vi "Mixed Mode Widget.vi"() -> ()   [LabVIEW 2009]
uses:
  lib/MixedMode/Mixed Mode Command Action.ctl
  lib/MixedMode/Target Data.ctl
  lib/MixedMode/Ramp Time Tuple.ctl
  lib/MixedMode/Messages/Mixed Mode Command.ctl
  lib/MixedMode/Mixed Mode Cartesian Data.ctl
  lib/MixedMode/Mixed Mode Convergence Status.ctl
  lib/MixedMode/Mixed Mode States.ctl
  lib/MixedMode/Messages/Mixed Mode Status.ctl
  lib/MixedMode Widget/Mixed Mode Widget Button States.ctl
  lib/MixedMode/Step DAO Actions.ctl
  lib/MixedMode Widget/NTCP MM Requests.ctl
  lib/MixedMode/Messages/Mixed Mode Button Events.ctl
  lib/Data Access Objects/Metadata/LBCB Number.ctl
  lib/MixedMode/Messages/Target.ctl
  lib/MixedMode/Messages/Mixed Mode Button Events Message.ctl
  lib/MixedMode/Messages/MM Widget Parameter Changes.ctl
  lib/Apps/GUI Control.ctl
  lib/MixedMode/Messages/Mixed Mode GUI Update Type.ctl
  lib/MixedMode/Messages/Mixed Mode Gui Update Msg.ctl
  lib/Global Data/Names/Name Actions.ctl
  lib/MixedMode/MCL States.ctl
  lib/MixedMode Widget/Manual States.ctl
  lib/MixedMode Widget/Input File Step Actions.ctl
  lib/MixedMode Widget/Input File States.ctl
  lib/Apps/Yes No Button.ctl
  NTCP library/NTCP Commands.ctl
  lib/NTCP Client/MM 2 NTCP Message.ctl
  lib/NTCP Client/NTCP 2 MM Message.ctl
  lib/Data Access Objects/Metadata/Persistant DAO Actions.ctl
  lib/MixedMode Widget/NTCP Mixed Mode States.ctl
  lib/Launcher/Launcher Actions.ctl
  lib/Launcher/NoPanelAppTypes.ctl
  lib/MixedMode Widget/Skip NTCP Close Monitor.ctl
  lib/MixedMode Widget/Run Or Stop Result.ctl
  lib/Apps/On Off Button.ctl
  lib/MixedMode Widget/Blinkies.ctl
  lib/Data Access Objects/Metadata/DAO Actions.ctl
  lib/MixedMode/Mixed Mode Archived State.ctl
  lib/IPC Messages/Offset Message Type.ctl
  lib/MixedMode Widget/Mixed Mode State Display.ctl
  lib/MixedMode Widget/Target Pattern.ctl
  lib/Data Display/External Sensor Name & Value.ctl
panel:
  out "Force Tag":string
  in  "Force Tags":string[](array[string])
  out "Typo Problem":bool
  out "Increment Limit":bool caption="Increment"
  out "From Queue":string
  out "To Queue":string
  out "NTCP":T1
  out "MCL States":T5
  out "NTCP MM Requests":T6
  out "Force Limit":bool caption="Force"
  out "Displacement Limit":bool caption="Displacement"
  out "Messages":string
  out "Mixed Mode Status":T7={"LBCB Target"=[], "MixedModeStates"=enum."Idle", "LBCB Convergence"=[], "LBCB Measurements"=[]}
  in  "App Running":bool
  out "Button States":T12
  in  "App Stop":bool
  out "Mixed Mode Command":T13
  in  "Cartesian Type":bool caption="CartesianType"
  in  "Channel Data Tables":T16(tab)
  in  "LBCB 2 Label":string="LBCB 2"
  out "Cartesian Labels L1":string[](array[string])=["X", "Y", "Z", "Rx", "Ry", "Rz"]
  out "LBCB 1 Cartesian Space":dbl[][](array[numeric]) caption="LBCB 1"
  out "LBCB 2 Cartesian Space":dbl[][](array[numeric]) caption="LBCB 2"
  out "Cartesian Labels L2":string[](array[string])=["X", "Y", "Z", "Rx", "Ry", "Rz"]
  out "Cartesian Space Labels":string[](array[string])=["Commands (in/rad)", "Displacements (in/rad)", "Forces (lbs/lb*in)"]
  in  "LBCB 1 Label":string="LBCB 1"
  out "Actuator Labels L2":string[](array[string])=["X1", "X2", "Y1", "Z1", "Z2", "Z3"]
  out "LBCB 2 Actuator Space":dbl[][](array[numeric]) caption="LBCB 2"
  out "LBCB 1 Actuator Space":dbl[][](array[numeric]) caption="LBCB 1"
  out "Actuator Labels L1":string[](array[string])=["X1", "X2", "Y1", "Z1", "Z2", "Z3"]
  out "Actuator Space Labels":string[](array[string])=["Commands (in)", "Displacements (in)", "Forces (lbs)", "Integral"]
  out "External Sensors":T17[](array[typedef])
  out "Test Statistics":cluster{"Steps":string, "Elapsed \nTime":dbl} {"Elapsed \nTime" format="%<%H:%M:%S>t"}
  in  "Mixed Mode Control Tabs":enum32{"Manual", "Input File", "NTCP"}(tab)
  in  "Set Target":bool
  in  "Target Pattern":T18
  in  "Apply Pattern":bool
  out "Manual States":T19
  in  "Run Infile":bool
  out "Running":bool
  in  "Reset":bool
  in  "Load File":bool
  out "Input File States":T20
  in  "Connect Server":bool
  in  "Control Point":string="MDL-00-01"
  out "Connected":bool
  out "NTCP MM States":T21
  in  "Execute":cluster{"Auto":bool, "Start":bool, "Stop":bool}
  in  "Propose":T22
  out "Mixed Mode State Display":T23
  out "Current Values":T3[](array[typedef])
  in  "Ramp Times":cluster{"Displacement":T15, "Force":T15}={"Displacement"={"Ramp"=5.0, "Stab"=4.0, "Hold"=5.0}, "Force"={"Ramp"=5.0, "Stab"=4.0, "Hold"=5.0}}
  in  "Targets":T3[](array[typedef])
  # "Limit\nFaults"
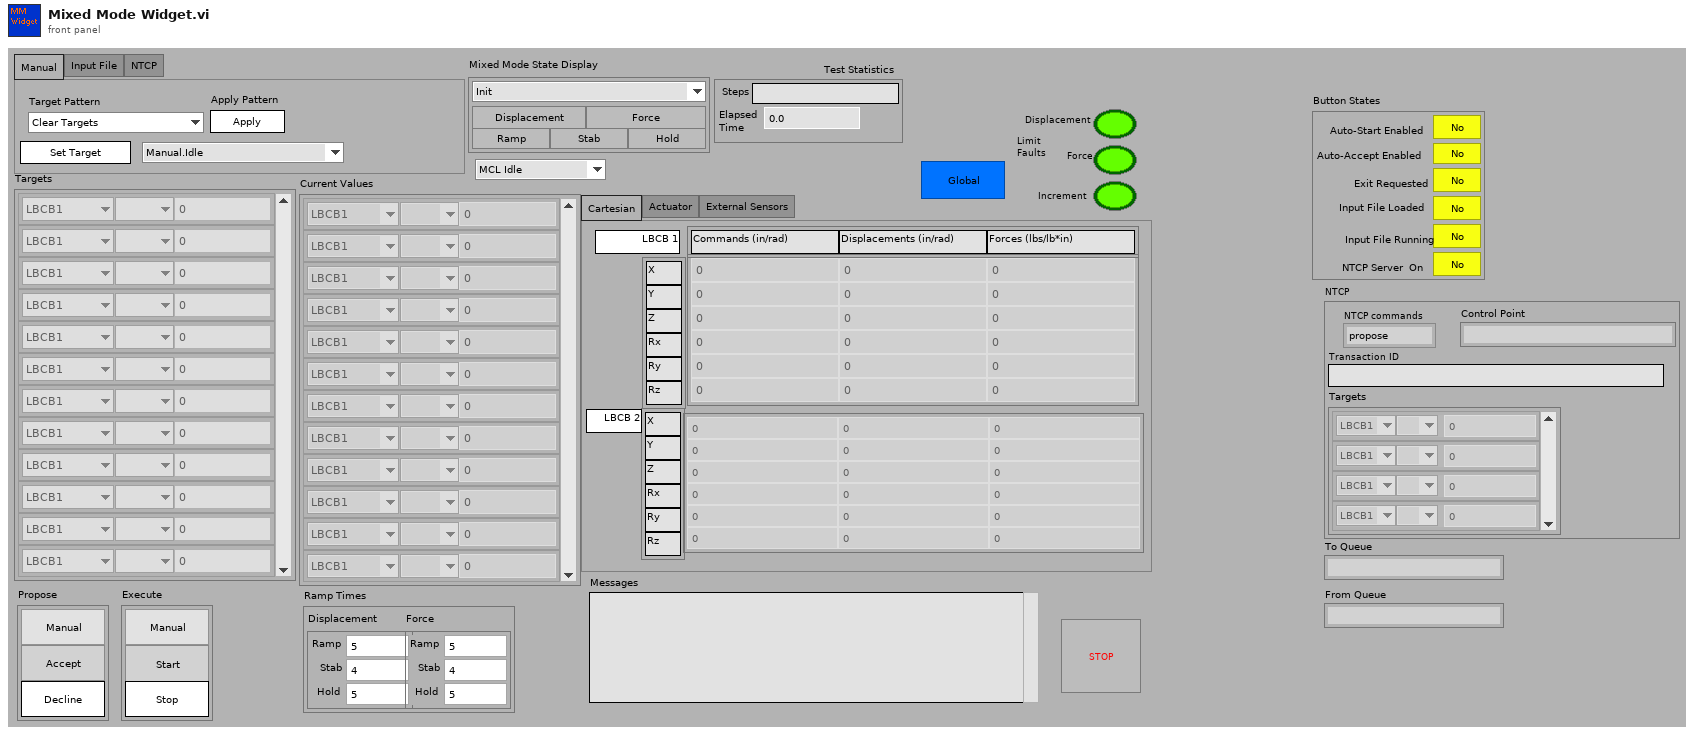
[diagram p1: front panel]
types:
  T1 = typedef "NTCP 2 MM Message.ctl" = cluster{"NTCP commands":T2, "Transaction ID":string, "Control Point":string, "Targets":T3[]}
  T2 = typedef "NTCP Commands.ctl" = enum16{"propose", "execute", "cancel", "set-parameter", "get-parameter", "open-session", "close-session", "get-control-point", "Unknown", "stop"}
  T3 = typedef "Target.ctl" = cluster{"LBCB Number":T4, "DOF Vectors":enum16{" ", "Dx", "Dy", "Dz", "Rx", "Ry", "Rz", "Fx", "Fy", "Fz", "Mx", "My", "Mz"}, "Amount":dbl}
  T4 = typedef "LBCB Number.ctl" = enum16{"LBCB1", "LBCB2"}
  T5 = typedef "MCL States.ctl" = enum16{"MCL Idle", "MCL Ramping", "MCL Holding", "MCL Aborting", "MCL Done", "MCL NOP"}
  T6 = typedef "NTCP MM Requests.ctl" = cluster{"Execute Pending":bool, "Propose Pending":bool, "Connected":bool, "Reset":bool}
  T7 = typedef "Mixed Mode Status.ctl" = cluster{"LBCB Target":T8[], "MixedModeStates":T9, "LBCB Convergence":T10[], "LBCB Measurements":T11[]}
  T8 = typedef "Target Data.ctl" = cluster{"Displacements":dbl[], "Command Type":enum16{"<None>", "Displacement", "Force"}[], "Forces":dbl[]}
  T9 = typedef "Mixed Mode States.ctl" = enum16{"Init", "Wait For DAQ", "Idle", "Start Initial Position", "Initial Position", "Start Initial Ramp", "Run Initial Ramp", "Start Iterative Stage", "Convergence Check", "Update Stiffness Jacobian", "Update Command", "Start Iterative Ramp", "Run Iterative Ramp", "Start Iterative Stabilize", "Iterative Stabilize", "Start Iterative Holding", "Iterative Holding", "Start Stabilize", "Stabilize", "Start Hold", "Holding", "Done", "Aborting", "Exit", "Nop"}
  T10 = typedef "Mixed Mode Convergence Status.ctl" = cluster{"IsConverged":bool[], "Force Errors":dbl[], "Controlling DOF":bool[]}
  T11 = typedef "Mixed Mode Cartesian Data.ctl" = cluster{"Displacements":dbl[], "Forces":dbl[]}
  T12 = typedef "Mixed Mode Widget Button States.ctl" = cluster{"Auto-Start Enabled":bool, "Auto-Accept Enabled":bool, "Exit Requested":bool, "Input File Loaded":bool, "Input File Running":bool, "NTCP Server  On":bool}
  T13 = typedef "Mixed Mode Command.ctl" = cluster{"Command":T14, "Ramp Times":cluster{"Initial":T15, "Iterative":T15}, "LBCB1":T8, "LBCB2":T8}
  T14 = typedef "Mixed Mode Command Action.ctl" = enum16{"Start Command", "Stop", "Exit", "No Op", "Start Acquisition", "Measure Initial Position"}
  T15 = typedef "Ramp Time Tuple.ctl" = cluster{"Ramp":dbl, "Stab":dbl, "Hold":dbl}
  T16 = enum32{"Cartesian", "Actuator", "External Sensors"}
  T17 = typedef "External Sensor Name & Value.ctl" = cluster{"Name":string, "Value":dbl}
  T18 = typedef "Target Pattern.ctl" = enum16{"Clear Targets", "Reset Targets to Zero", "Displacements Only", "Rotations Only", "Displacements & Rotations", "Forces Only", "Moments Only", "Forces & Moments"}
  T19 = typedef "Manual States.ctl" = enum16{"Manual.Idle", "Manual.WaitForStart", "Manual.WaitForMclRamp", "Manual.WaitForMclDone", "Manual.Abort", "Manual.InitialPosition"}
  T20 = typedef "Input File States.ctl" = enum16{"InputFile.Idle", "InputFile.WaitForRunning", "InputFile.StepsAvailable", "InputFile.LoadStep", "InputFile.WaitForAccept", "InputFile.WaitForStart", "InputFile.WaitForMclRamp", "InputFile.WaitForMclDone", "InputFile.StopRunning"}
  T21 = typedef "NTCP Mixed Mode States.ctl" = enum16{"Ntcp.Off", "Ntcp.WaitForProposal", "Ntcp.WaitForAccept", "Ntcp.WaitForExecute", "Ntcp.WaitForStart", "Ntcp.WaitForMclRamp", "Ntcp.WaitForMclDone", "Ntcp.Shutdown"}
  T22 = cluster{"Auto":bool, "Accept":bool, "Decline":bool}
  T23 = typedef "Mixed Mode State Display.ctl" = cluster{"MixedModeStates":T9, "Initial":bool, "Iterative":bool, "Ramp":bool, "Stab":bool, "Hold":bool}
  T24 = typedef "DAO Actions.ctl" = enum16{"Init", "Get", "Set"}
  T25 = typedef "Mixed Mode Archived State.ctl" = cluster{"MixedModeStates":T9, "Step":string}
  T26 = typedef "MM 2 NTCP Message.ctl" = cluster{"NTCP commands":T2, "Transaction ID":string, "Control Point":string, "Accepted":T27}
  T27 = typedef "Yes No Button.ctl" = bool
  T28 = typedef "Blinkies.ctl" = cluster{"Accept":T29, "Start":T29}
  T29 = typedef "On Off Button.ctl" = bool
  T30 = typedef "Name Actions.ctl" = enum16{"Init", "Get Names", "Get Index"}
  T31 = typedef "Mixed Mode Gui Update Msg.ctl" = cluster{"MM GUI Update Type":T32, "Targets":T3[], "State":bool, "Step":string}
  T32 = typedef "Mixed Mode GUI Update Type.ctl" = enum16{"Nop", "Targets", "Accept.Blink", "Start.Blink", "TestStats", "Control.Enabled", "StartTestTimer", "RunInputFile", "NTCP Server", "Propose.Auto", "Execute.Auto", "All Autos Off", "Input File Loaded", "Exit"}
  T33 = typedef "GUI Control.ctl" = cluster{"Command":T34, "LBCB Number":enum16{"LBCB1", "LBCB2"}}
  T34 = typedef "MM Widget Parameter Changes.ctl" = enum16{"Start", "Stop All", "Control Enabled", "Control Disabled"}
  T35 = typedef "Mixed Mode Button Events Message.ctl" = cluster{"MM Control Events":T36, "Button States":T12}
  T36 = typedef "Mixed Mode Button Events.ctl" = enum16{"Propose.Accept", "Propose.Decline", "Execute.Start", "Execute.Stop", "TargetSet", "InputFile.Load", "InputFile.Reset", "InputFile.Pause", "InputFile.Run", "CartesianType.Changed", "NCTP.ConnectToServer", "NTCP.DisconnectFromServer", "Application.Stop", "Control.Enabled", "Control.Disabled", "ControlType.Changed", "Nop", "Manual.SetInitialPosition"}
  T37 = typedef "Persistant DAO Actions.ctl" = enum16{"Init", "Get", "Set", "Load", "Save"}
  T38 = enum16{"Init", "Set Step", "Set Correction Step", "Set Step String", "Get Step String"}
  T39 = typedef "Step DAO Actions.ctl" = enum16{"Init", "Set", "Get", "Reset Count"}
  T40 = typedef "Offset Message Type.ctl" = cluster{"Cartesian Type":bool, "Force Tag":string}
  T41 = typedef "Number Of LBCBs.ctl" = enum16{"1", "2"}
  T42 = typedef "LBCB Settings.ctl" = cluster{"Size":T43, "Type":T44}
  T43 = typedef "LBCB Size.ctl" = enum16{"1/5th-scale LBCB", "Full-scale LBCB", "Portable LBCB", "Mid-Scale LBCB"}
  T44 = typedef "LBCB Type.ctl" = enum16{"X Actuators On The Left", "X Actuators On The Right"}
  T45 = typedef "Ramp Time Input.ctl" = cluster{"Directional":T46, "Iterative":T46}
  T46 = typedef "Ramp Control.ctl" = cluster{"Ramp":dbl, "Stabilize":dbl, "Hold":dbl}
  T47 = enum8{"Enabled", "Disabled", "Disabled and Grayed Out"}
  T48 = typedef "Input File Step Actions.ctl" = enum16{"Load", "Next Step", "Reset", "Get Step", "Backup"}
  T49 = typedef "Run Or Stop Result.ctl" = enum16{"Nevermind", "Run", "Stop"}
  T50 = typedef "Load Step.ctl" = cluster{"Step Number":u32, "Targets":T3[]}
  T51 = typedef "Accepted or Declined.ctl" = enum16{"No Decision Yet", "Accepted", "Declined", "Abort"}
  T52 = typedef "MCL Done Or Abort.ctl" = enum16{"Done", "Abort", "Still Running"}
  T53 = typedef "Stop Requests.ctl" = enum16{"Nothing", "Stop Requested", "Abort Requested"}
  T54 = typedef "Steps Type.ctl" = cluster{"Step":i32, "Substep":i32, "Correction Step":i32}
  T55 = typedef "App Parameters.ctl" = cluster{"Monitor Loop":T56, "Ramp Time":T56, "Log Loop":T56, "TCP to DAQ":T56, "Logging Directory":path, "Log File Size (MBytes)":i64, "Volt Logging Loop":T56, "2 LBCB Archiving Mode":bool}
  T56 = typedef "Timing Parameters.ctl" = cluster{"Interval":dbl, "Rate ":dbl}
  T57 = typedef "NoPanelAppTypes.ctl" = enum16{"NTCP Socket", "Data Archiving", "DAQ Link", "Control Loops", "Cmd Disp Diffs", "LBCB Data", "Limits", "Mixed Mode Widget", "Offsets", "Debug"}
  T58 = typedef "Launcher Actions.ctl" = enum16{"Launch", "Stop All", "Stop", "Kill", "Running?", "Init"}
  T59 = typedef "Skip NTCP Close Monitor.ctl" = enum16{"Skip Nothing", "Skip NTCP", "Skip Button Event"}
  T60 = typedef "Network Parameters.ctl" = cluster{"Port Number":u16, "Notification Name":string, "Wait For Notification Timeout":i32}
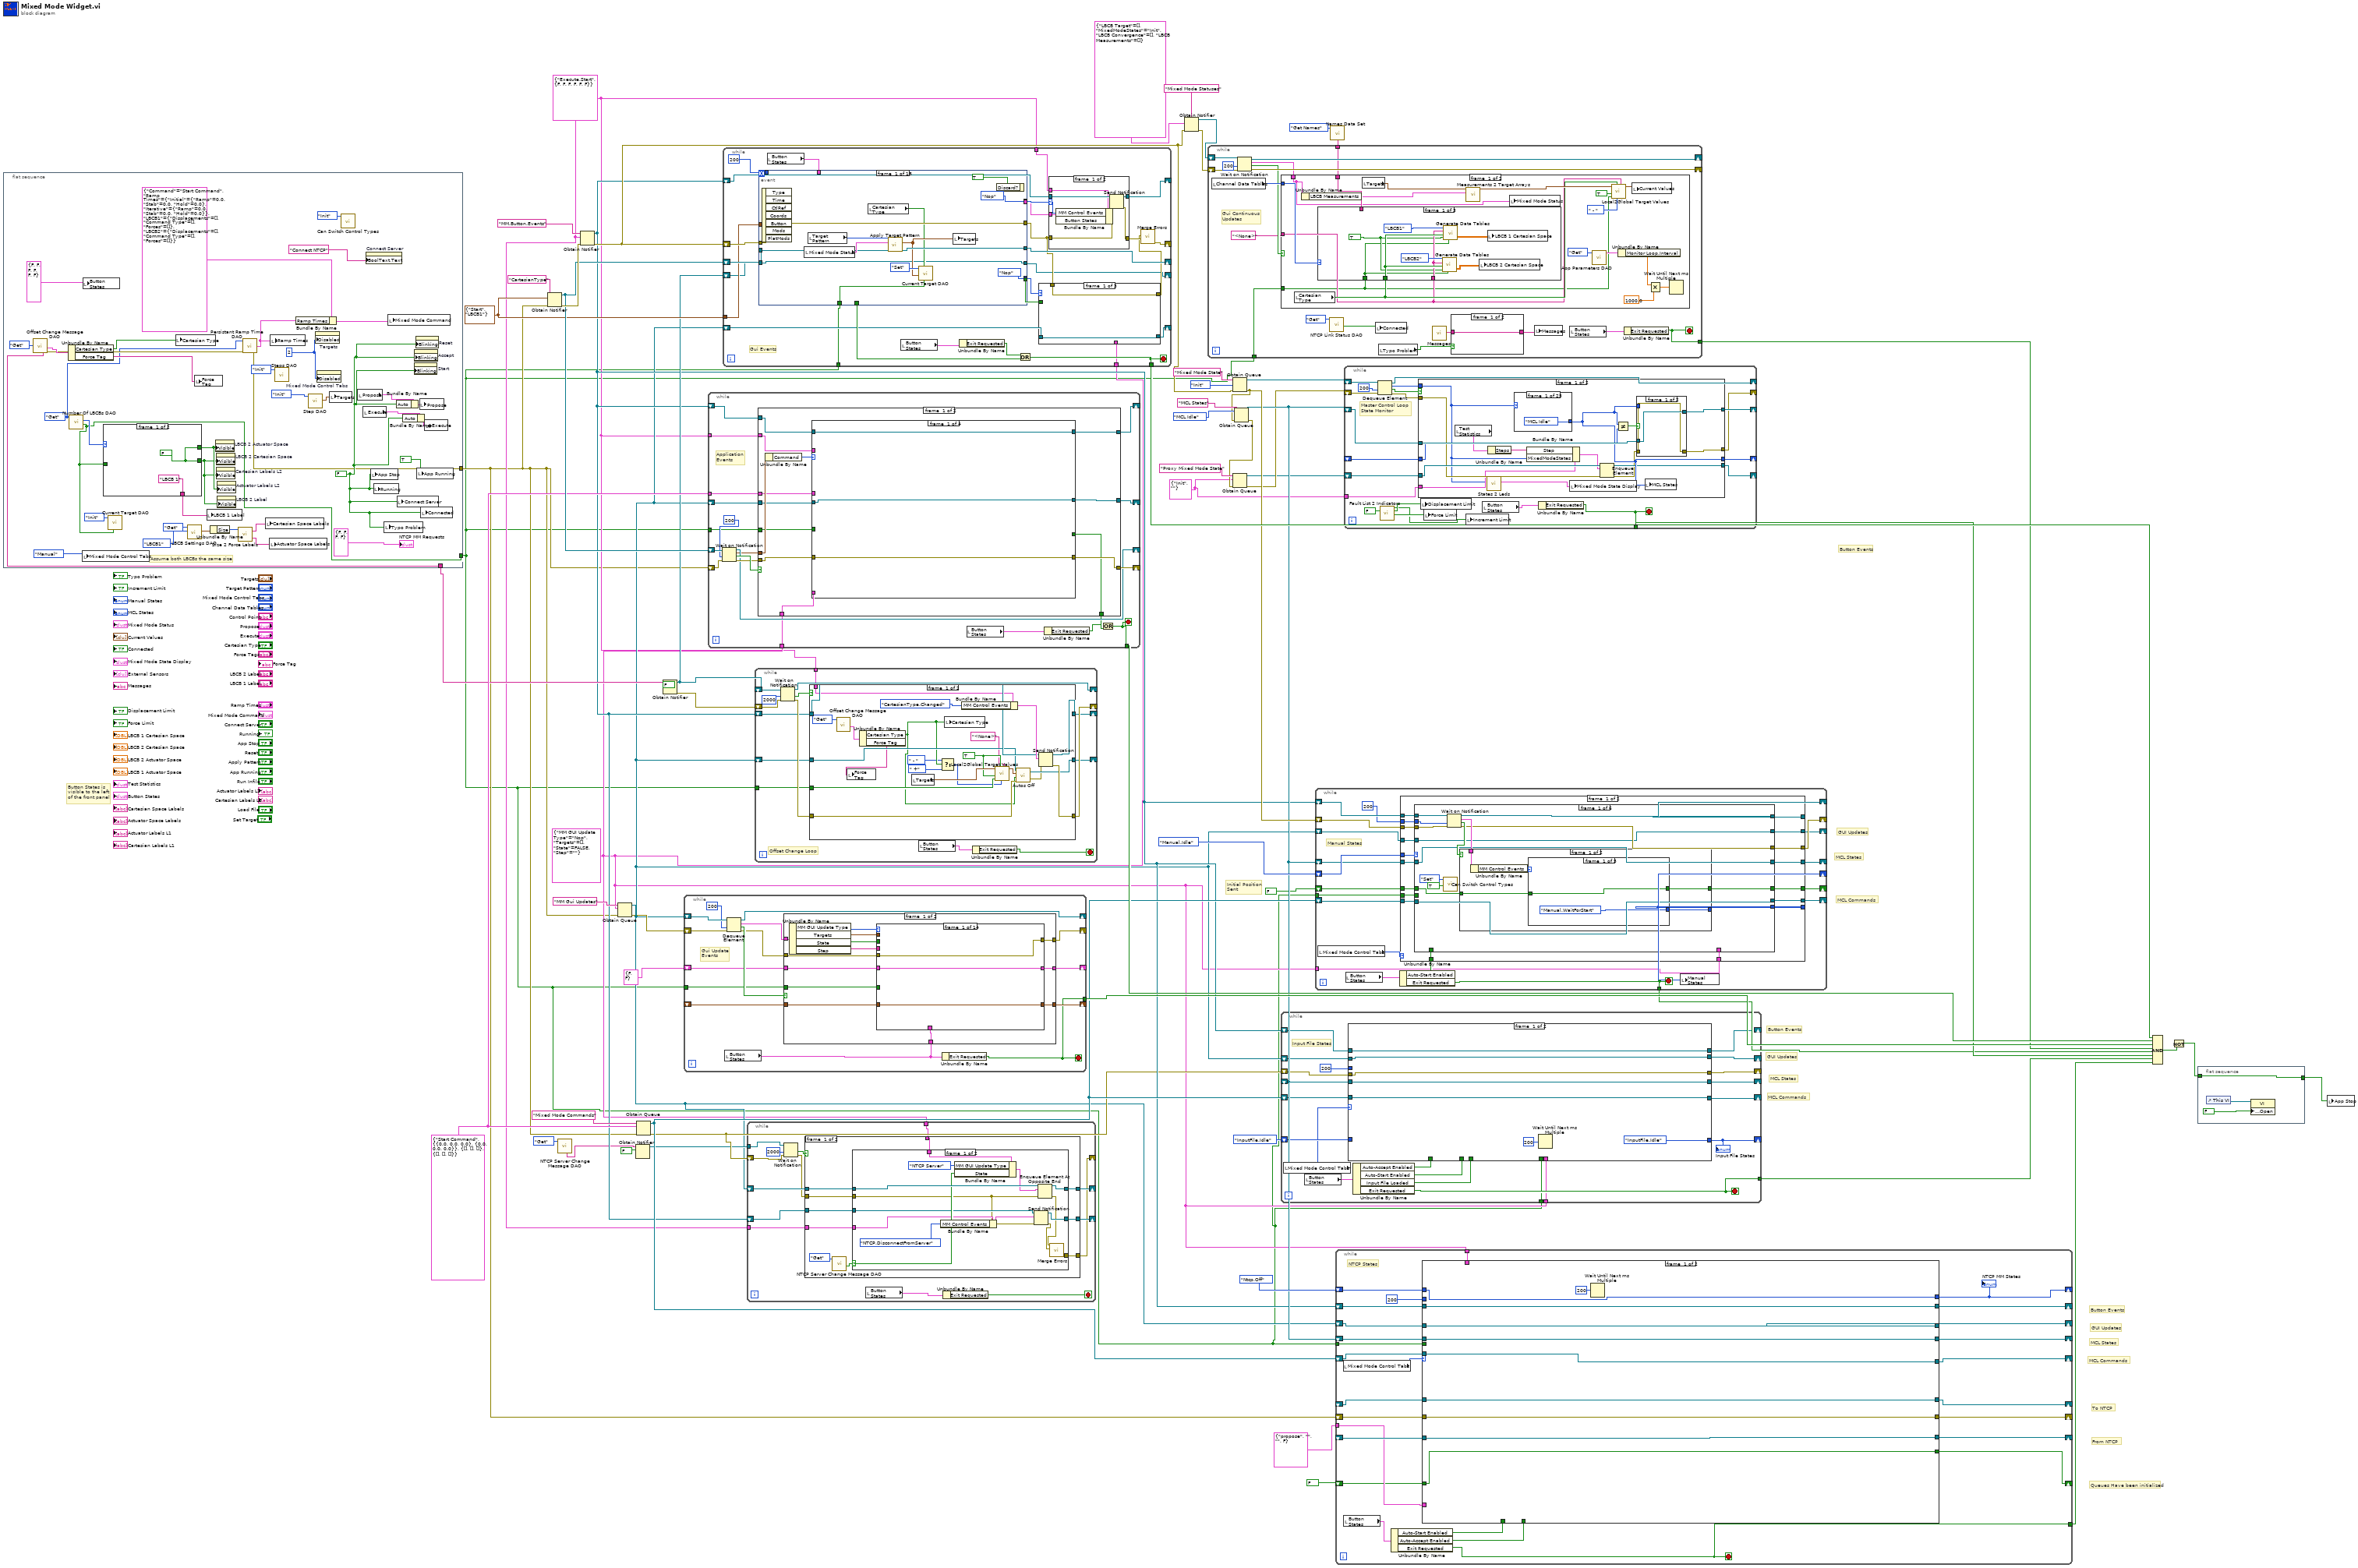
[diagram p0: block diagram]
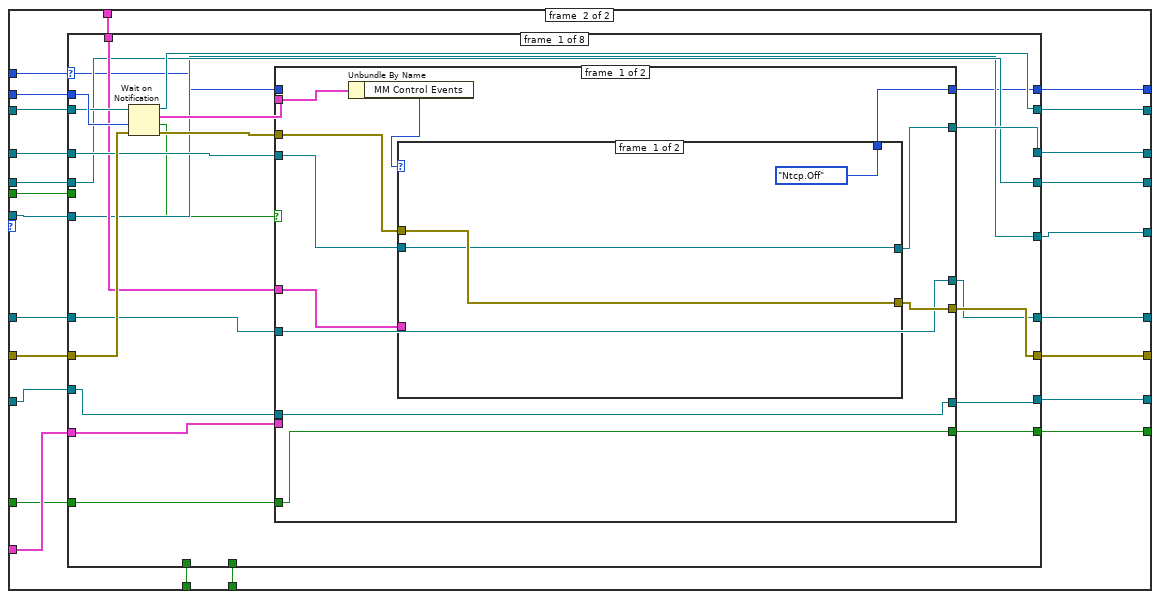
[diagram p5: hidden frame]
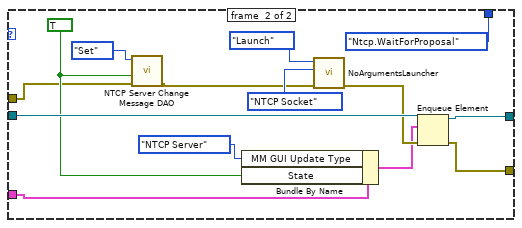
[diagram p6: hidden frame]
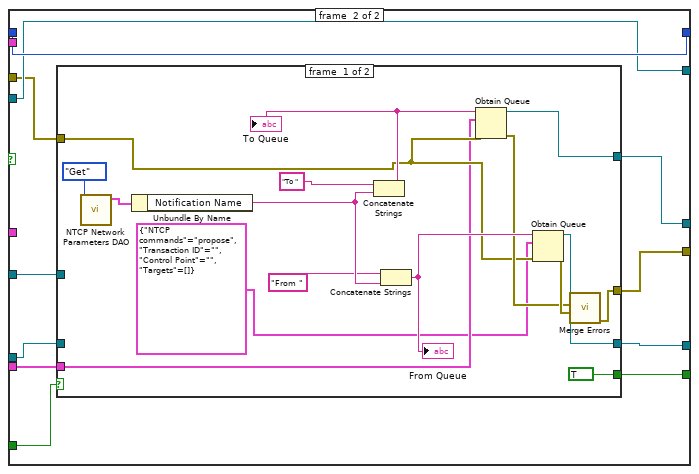
[diagram p7: hidden frame]
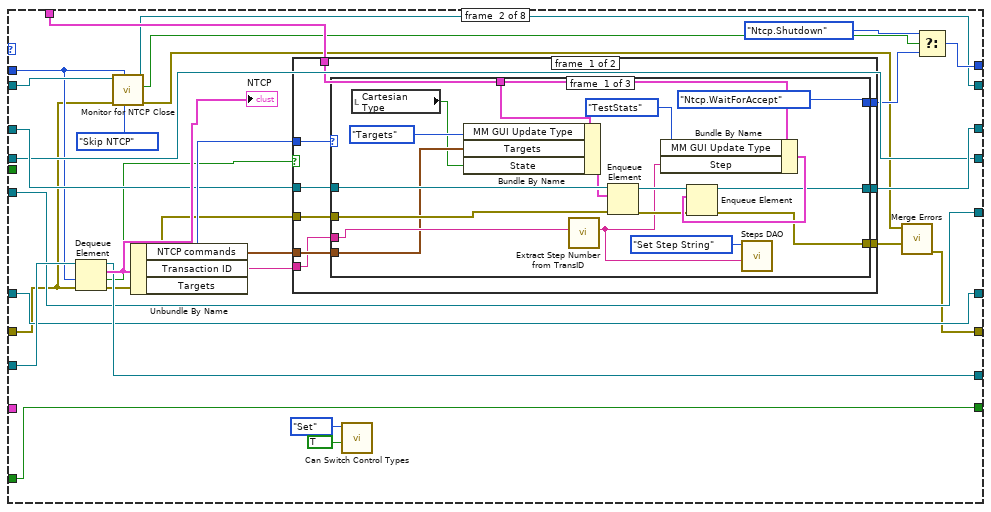
[diagram p9: hidden frame]
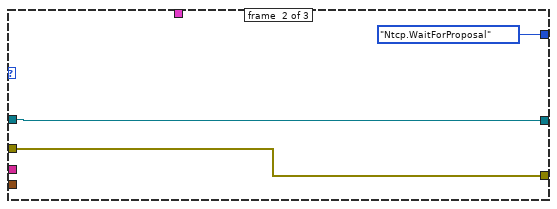
[diagram p10: hidden frame]
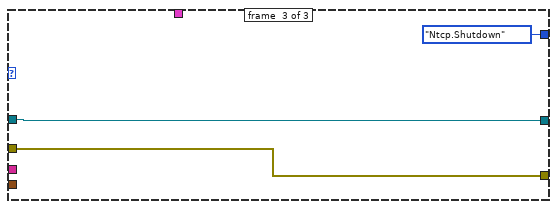
[diagram p11: hidden frame]
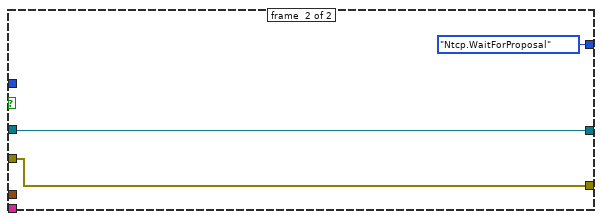
[diagram p12: hidden frame]
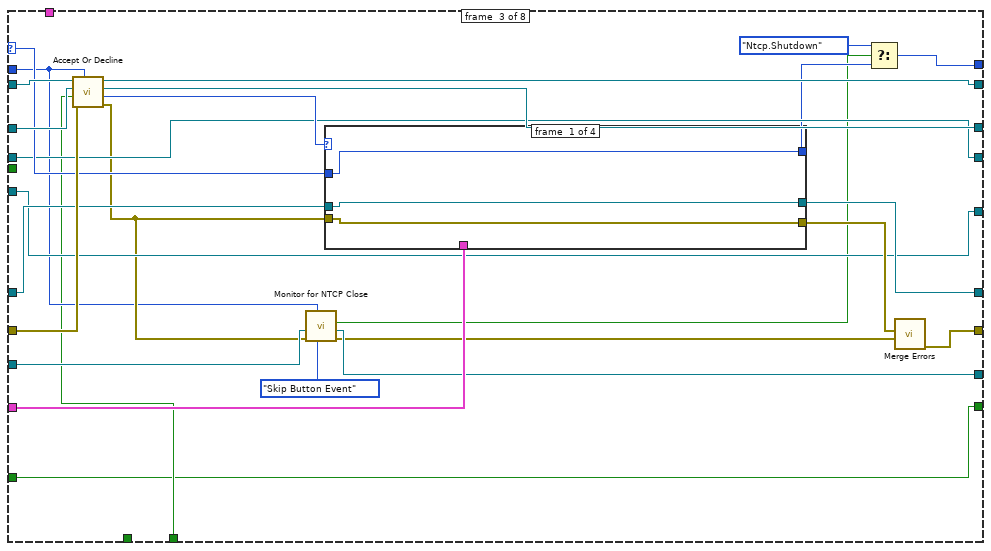
[diagram p13: hidden frame]
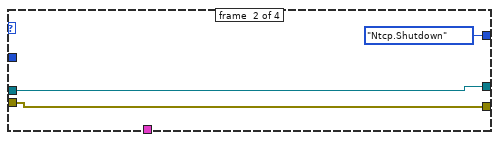
[diagram p14: hidden frame]
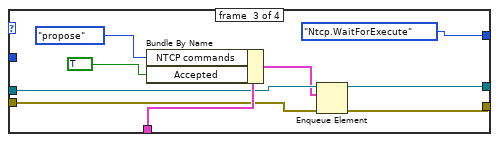
[diagram p15: hidden frame]
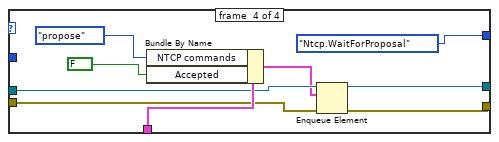
[diagram p16: hidden frame]
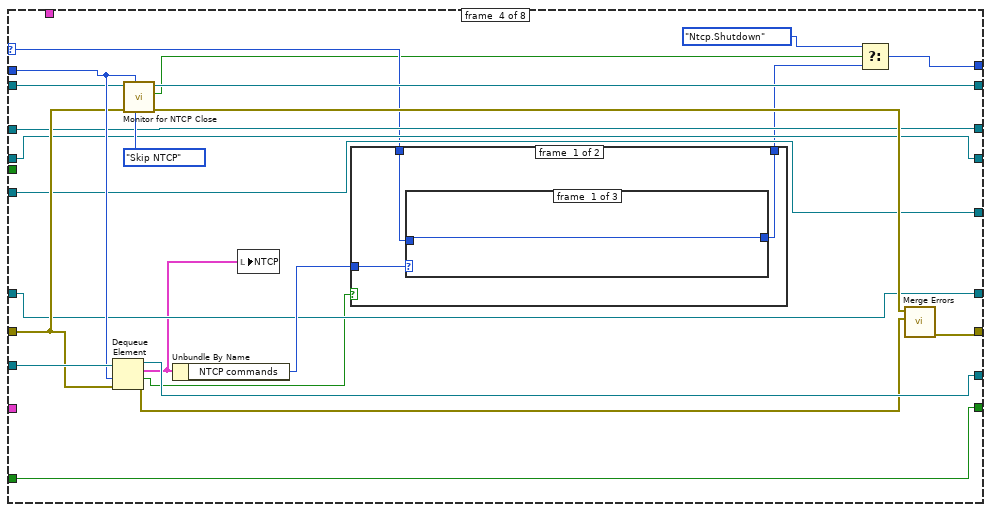
[diagram p17: hidden frame]
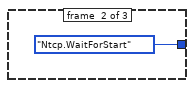
[diagram p18: hidden frame]
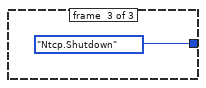
[diagram p19: hidden frame]
diagram:
  w17 = T25 {"MixedModeStates"=enum."Init", "Step"=""} ("Mixed Mode Archived State")
  w26 = T13 {"Command"=enum."Start Command", "Ramp Times"={"Initial"={"Ramp"=0.0, "Stab"=0.0, "Hold"=0.0}, "Iterative"={"Ramp"=0.0, "Stab"=0.0, "Hold"=0.0}}, "LBCB1"={"Displacements"=[], "Command Type"=[], "Forces"=[]}, "LBCB2"={"Displacements"=[], "Command Type"=[], "Forces"=[]}} ("Mixed Mode Command In")
  w5 = T31 {"MM GUI Update Type"=enum."Nop", "Targets"=[], "State"=FALSE, "Step"=""} ("MM Gui Update Msg")
  w28 = T33 {"Command"=enum."Start", "LBCB Number"=enum."LBCB1"} ("GUI Control")
  w4 = T35 {"MM Control Events"=enum."Execute.Start", "Button States"={"Auto-Start Enabled"=FALSE, "Auto-Accept Enabled"=FALSE, "Exit Requested"=FALSE, "Input File Loaded"=FALSE, "Input File Running"=FALSE, "NTCP Server  On"=FALSE}} ("MM Button Events Msg")
  # "Initial Position\nSent"
  # "Button States is \nvisible to the left\nof the front panel"
  # "Queues Have been initialized"
  # "Button Events"
  # "GUI Updates"
  # "MCL States"
  # "MCL Commands"
  # "From NTCP"
  # "To NTCP"
  # "Button Events"
  # "GUI Updates"
  # "MCL States"
  # "MCL Commands"
  # "Button Events"
  # "GUI Updates"
  # "MCL States"
  # "MCL Commands"
  n1 = flat-sequence {
    tunnel: [w71] -> w3
    tunnel: [w63] -> w2
    tunnel: [w70] -> w15
    frame #0 {
      w65 = Persistant_DAO_Actions."Get" ("Actions")
      w91 = u8 2 ("Disabled")
      w85 = FALSE ("Exit")
      # "Assume both LBCBs the same size"
      n2 = call "Offset Change Message DAO.vi"("DAO Actions"=DAO_Actions."Get") -> ("error out"=w71:errorcluster, "Offset Out"=w72:T40, "Notifier Name"=w70:string)  [unwired: 8 in]
      n3 = Unbundle By Name(w72) -> ("Cartesian Type"=w69:bool, "Force Tag"=w66:string)
      n4 = call "Number Of LBCBs DAO.vi"("Actions"=w65) -> ("Rigid Connection Out"=w63:bool, "Number of\nLBCBs Out"=w77:T41)  [unwired: 7 in, 2 out]
      n5 = local write "Mixed Mode Control Tabs"(enum32{"Manual", "Input File", "NTCP"}."Manual" ("Mixed Mode Control Tabs")) -> ()
      n6 = local write "Button States"(T12 {"Auto-Start Enabled"=FALSE, "Auto-Accept Enabled"=FALSE, "Exit Requested"=FALSE, "Input File Loaded"=FALSE, "Input File Running"=FALSE, "NTCP Server  On"=FALSE} ("Mixed Mode Widget Requests")) -> ()
      n7 = case shown="\"2\"" w77 {
        tunnel: [w100 w105] -> w74
        tunnel: w63 -> [_ w104]
        tunnel: ["LBCB 1" w103] -> w76
        tunnel: [w100 TRUE] -> w75
        frame #0 {
          w100 = FALSE
        }
        frame #1 {
          n8 = case shown="True" w104 {
            tunnel: [TRUE FALSE] -> w105
            tunnel: ["LBCB 1" "Combined"] -> w103
            frame #0 {
            }
            frame #1 {
            }
          }
        }
      }
      n9 = call "Current Target DAO.vi"("Combined"=w63, "DAO Actions"=DAO_Actions."Init") -> ()  [unwired: 8 in, 2 out]
      n10 = local write "Cartesian Type"(w69) -> ()
      n11 = call "LBCB Settings DAO.vi"("LBCB Number"=LBCB_Number."LBCB1", "Actions"=Persistant_DAO_Actions."Get") -> ("LBCB Setting Out"=w81:T42)  [unwired: 7 in, 2 out]
      n12 = local write "Force Tag"(w66) -> ()
      n13 = local write "LBCB 1 Label"(w76) -> ()
      n14 = Unbundle By Name(w81) -> ("Size"=w80:T43)
      n15 = property on="LBCB 2 Actuator Space" class="Arr (strict)"("Visible"=w75) -> ()  [unwired: 2 in, 2 out]
      n16 = property on="LBCB 2 Cartesian Space" class="Arr (strict)"("Visible"=w74) -> ()  [unwired: 2 in, 2 out]
      n17 = property on="Cartesian Labels L2" class="Arr (strict)"("Visible"=w74) -> ()  [unwired: 2 in, 2 out]
      n18 = property on="Actuator Labels L2" class="Arr (strict)"("Visible"=w75) -> ()  [unwired: 2 in, 2 out]
      n19 = property on="LBCB 2 Label" class="Str"("Visible"=w74) -> ()  [unwired: 2 in, 2 out]
      n20 = call "Size 2 Force Labels.vi"("Size"=w80) -> ("Actuator Space Labels"=w78:string[], "Cartesian Space Labels In"=w79:string[])  [unwired: 1 in]
      n21 = call "Persistant Ramp Time DAO.vi"("Ramp Time Actions"=w65) -> ("Ramp Time Out"=w64:T45)  [unwired: 3 in, 11 out]
      n22 = local write "Cartesian Space Labels"(w79) -> ()
      n23 = local write "Actuator Space Labels"(w78) -> ()
      n24 = local write "Ramp Times"(w64) -> ()
      n25 = call "Steps DAO.vi"("Steps Actions"=T38."Init") -> ()  [unwired: 8 in, 3 out]
      n26 = Bundle By Name(cluster=T13 {"Command"=enum."Start Command", "Ramp Times"={"Initial"={"Ramp"=0.0, "Stab"=0.0, "Hold"=0.0}, "Iterative"={"Ramp"=0.0, "Stab"=0.0, "Hold"=0.0}}, "LBCB1"={"Displacements"=[], "Command Type"=[], "Forces"=[]}, "LBCB2"={"Displacements"=[], "Command Type"=[], "Forces"=[]}} ("Mixed Mode Command"), "Ramp Times"=w64) -> (w89:T13)
      n27 = call "Step DAO.vi"("Step DAO Actions"=Step_DAO_Actions."Init") -> ("Step Out"=w98:T3[])  [unwired: 3 in, 7 out]
      n28 = property on="Targets" class="Arr (strict)"("Disabled"=w91) -> ()  [unwired: 2 in, 2 out]
      n29 = property on="Mixed Mode Control Tabs" class="TabCtl (strict)"("Disabled"=w91) -> ()  [unwired: 2 in, 2 out]
      n30 = local write "Targets"(w98) -> ()
      n31 = call "Can Switch Control Types.vi"("DAO Actions"=DAO_Actions."Init") -> ()  [unwired: 10 in, 1 out]
      n32 = local read "Propose"() -> (w94:T22)
      n33 = local read "Execute"() -> (w92:cluster{"Auto":bool, "Start":bool, "Stop":bool})
      n34 = property on="Connect Server" class="Bool (strict)"("BoolText.Text"="Connect NTCP" ("Boolean Text.Text")) -> ()  [unwired: 2 in, 2 out]
      n35 = local write "App Stop"(w85) -> ()
      n36 = local write "Running"(w85) -> ()
      n37 = local write "Typo Problem"(w85) -> ()
      n38 = local write "Mixed Mode Command"(w89) -> ()
      n39 = Bundle By Name(cluster=w94, "Auto"=w85) -> (w95:T22)
      n40 = local write "Connect Server"(w85) -> ()
      n41 = Bundle By Name(cluster=w92, "Auto"=w85) -> (w93:cluster{"Auto":bool, "Start":bool, "Stop":bool})
      n42 = property on="Start" class="Bool (strict)"("Blinking"=w85) -> ()  [unwired: 2 in, 2 out]
      n43 = property on="Accept" class="Bool (strict)"("Blinking"=w85) -> ()  [unwired: 2 in, 2 out]
      n44 = property on="Reset" class="Bool"("Blinking"=w85) -> ()  [unwired: 2 in, 2 out]
      n45 = local write "App Running"(TRUE) -> ()
      n46 = local write "Propose"(w95) -> ()
      n47 = local write "Connected"(w85) -> ()
      n48 = local write "Execute"(w93) -> ()
      "NTCP MM Requests" <- T6 {"Execute Pending"=FALSE, "Propose Pending"=FALSE, "Connected"=FALSE, "Reset"=FALSE} ("NTCP MM Requests")
    }
  }
  n49 = Obtain Notifier(name (unnamed)="CartesianType", notification data type=w28, error in (no error)=w3) -> (notifier out=w29:refnum<notifier>, error out=w57:errorcluster)  [unwired: 1 in, 1 out]
  n50 = call "NTCP Server Change Message DAO.vi"("DAO Actions"=DAO_Actions."Get") -> ("Notifier Name"=w7:string)  [unwired: 8 in, 2 out]
  n51 = Obtain Notifier(name (unnamed)="MM.Button.Events", notification data type=w4, error in (no error)=w57) -> (notifier out=w12:refnum<notifier>, error out=w43:errorcluster)  [unwired: 1 in, 1 out]
  n52 = Obtain Queue(name (unnamed)="MM Gui Updates", element data type=w5, error in (no error)=w3) -> (queue out=w6:refnum<queue>, error out=w53:errorcluster)  [unwired: 2 in, 1 out]
  n53 = Obtain Notifier(name (unnamed)=w7, notification data type=FALSE) -> (notifier out=w9:refnum<notifier>)  [unwired: 2 in, 2 out]
  n54 = Obtain Queue(name (unnamed)="Mixed Mode Commands", element data type=w26, error in (no error)=w3) -> (queue out=w27:refnum<queue>, error out=w10:errorcluster)  [unwired: 2 in, 1 out]
  n55 = Obtain Notifier(name (unnamed)=w15, notification data type=FALSE) -> (notifier out=w14:refnum<notifier>, error out=w13:errorcluster)  [unwired: 2 in, 1 out]
  n56 = while {
    shift-right: [w117] -> _
    shift-left: w53 -> [w122]
    shift-right: [w121] -> _
    shift-left: w6 -> [w124]
    shift-right: [w116] -> _
    shift-left: _ -> [w115]
    tunnel: [w114] -> w52
    shift-right: [w111] -> _
    shift-left: T28 {"Accept"=FALSE, "Start"=FALSE} ("Blinkies") -> [w112]
    tunnel: w2 -> [w110]
    stop <- w114 stop-if-true
    # "Gui Update\nEvents"
    n57 = local read "Button States"() -> (w113:T12)
    n58 = Dequeue Element(queue=w124, timeout in ms (-1)=200, error in (no error)=w122) -> (queue out=w121:refnum<queue>, element=w120:T31, timed out?=w119:bool, error out=w118:errorcluster)
    n59 = case shown="False" w119 {
      tunnel: w120 -> [w137 _]
      tunnel: w118 -> [w133 w240]
      tunnel: [w132 w240] -> w117
      tunnel: [w130 w239] -> w116
      tunnel: w115 -> [w129 w239]
      tunnel: w113 -> [w128 _]
      tunnel: w112 -> [w127 w238]
      tunnel: [w126 w238] -> w111
      tunnel: w110 -> [w125 _]
      frame #0 {
        n60 = Unbundle By Name(w137) -> ("MM GUI Update Type"=w136:T32, "Targets"=w135:T3[], "State"=w134:bool, "Step"=w131:string)
        n61 = case shown="\"Targets\"" w136 {
          tunnel: w135 -> [_ _ w146 _ _ _ _ _ _ _ _ _ _ _]
          tunnel: w134 -> [_ _ w144 w152 w164 _ w184 w189 w200 _ w216 w221 w230 _]
          tunnel: w133 -> [w140 w143 w149 w158 w170 w177 w188 w197 w203 w209 w214 w220 w228 w236]
          tunnel: [w140 w143 w149 w157 w169 w177 w188 w197 w203 w209 w212 w220 w228 w236] -> w132
          tunnel: w131 -> [_ _ _ _ _ w175 _ _ _ _ _ _ _ _]
          tunnel: [w139 w142 w150 w156 w168 w178 w186 w195 w198 w205 w211 w225 w233 w237] -> w130
          tunnel: w129 -> [w139 w142 w150 w156 w168 w178 _ _ w198 w205 w211 w225 w233 _]
          tunnel: w128 -> [_ _ _ _ _ _ w185 w194 w201 w207 _ w224 w232 _]
          tunnel: w127 -> [w138 w141 w148 w153 w165 w176 w187 w196 w202 w208 w210 w219 w227 w235]
          tunnel: [w138 w141 w148 w151 w163 w176 w187 w196 w202 w208 w210 w219 w227 w235] -> w126
          tunnel: w125 -> [_ _ w145 _ _ _ _ _ _ _ _ _ _ _]
          frame #0 {
          }
          frame #1 {
          }
          frame #2 {
            n62 = local write "Targets"(w146) -> ()
            n63 = call "Current Target DAO.vi"("Combined"=w145, "Use Offsets"=w144, "Targets In"=w146, "DAO Actions"=DAO_Actions."Set") -> ()  [unwired: 6 in, 2 out]
          }
          frame #3 {
            n64 = Unbundle By Name(w153) -> ("Start"=w154:T29)
            n65 = Not Equal?(x=w152, y=w154) -> (x != y?=w155:T29)
            n66 = case shown="False" w155 {
              tunnel: w158 -> [w159 w162]
              tunnel: w152 -> [_ w161]
              tunnel: [w159 w160] -> w157
              frame #0 {
              }
              frame #1 {
                n67 = property on="Start" class="Bool (strict)"(error in=w162, "Blinking"=w161) -> (error out=w160:errorcluster)  [unwired: 1 in, 1 out]
              }
            }
            n68 = Bundle By Name(cluster=w153, "Start"=w152) -> (w151:T28)
          }
          frame #4 {
            n69 = Unbundle By Name(w165) -> ("Accept"=w166:T29)
            n70 = Not Equal?(x=w164, y=w166) -> (x != y?=w167:T29)
            n71 = case shown="True" w167 {
              tunnel: w170 -> [w171 w174]
              tunnel: w164 -> [_ w173]
              tunnel: [w171 w172] -> w169
              frame #0 {
              }
              frame #1 {
                n72 = property on="Accept" class="Bool (strict)"(error in=w174, "Blinking"=w173) -> (error out=w172:errorcluster)  [unwired: 1 in, 1 out]
              }
            }
            n73 = Bundle By Name(cluster=w165, "Accept"=w164) -> (w163:T28)
          }
          frame #5 {
            n74 = Get Date/Time In Seconds() -> (seconds since 1Jan1904=w179:timestamp)
            n75 = Subtract(x=w179, y=w178) -> (x-y=w180:dbl)
            n76 = Bundle By Name(cluster=cluster{"Steps":string, "Elapsed \nTime":dbl} {"Steps"="", "Elapsed \nTime"=0.0} ("Test Statistics"), "Steps"=w175, "Elapsed \nTime"=w180) -> (w181:cluster{"Steps":string, "Elapsed \nTime":dbl})
            n77 = local write "Test Statistics"(w181) -> ()
          }
          frame #6 {
            n78 = Bundle By Name(cluster=w185, "Input File Running"=w184) -> (w183:T12)
            n79 = local write "Running"(w184) -> ()
            n80 = local write "Button States"(w183) -> ()
            n81 = Get Date/Time In Seconds() -> (seconds since 1Jan1904=w186:timestamp)
          }
          frame #7 {
            n82 = Bundle By Name(cluster=w194, "NTCP Server  On"=w189) -> (w193:T12)
            n83 = local write "Connect Server"(w189) -> ()
            n84 = local write "Button States"(w193) -> ()
            n85 = Select(t="Disconnect NTCP", s=w189, f="Connect NTCP" ("Boolean Text.Text")) -> (s? t:f=w192:string)
            n86 = property on="Connect Server" class="Bool (strict)"("BoolText.Text"=w192) -> ()  [unwired: 2 in, 2 out]
            n87 = Get Date/Time In Seconds() -> (seconds since 1Jan1904=w195:timestamp)
          }
          frame #8 {
            n88 = Bundle By Name(cluster=w201, "Input File Loaded"=w200) -> (w199:T12)
            n89 = local write "Button States"(w199) -> ()
          }
          frame #9 {
            n90 = Bundle By Name(cluster=w207, "Exit Requested"=TRUE) -> (w206:T12)
            n91 = local write "Button States"(w206) -> ()
          }
          frame #10 {
            n92 = Select(t=T47."Enabled" ("Disabled"), s=w216, f=T47."Disabled and Grayed Out" ("Disabled")) -> (s? t:f=w215:T47)
            n93 = property on="Mixed Mode Control Tabs" class="TabCtl (strict)"(error in=w214, "DisabledEnum"=w215) -> (error out=w213:errorcluster)  [unwired: 1 in, 1 out]
            n94 = property on="Targets" class="Arr (strict)"(error in=w213, "DisabledEnum"=w215) -> (error out=w212:errorcluster)  [unwired: 1 in, 1 out]
          }
          frame #11 {
            n95 = Bundle By Name(cluster=w224, "Auto-Accept Enabled"=w221) -> (w223:T12)
            n96 = Bundle By Name(cluster=T22 {"Auto"=FALSE, "Accept"=FALSE, "Decline"=FALSE} ("Propose"), "Auto"=w221) -> (w222:T22)
            n97 = local write "Button States"(w223) -> ()
            n98 = local write "Propose"(w222) -> ()
          }
          frame #12 {
            n99 = Bundle By Name(cluster=w232, "Auto-Start Enabled"=w230) -> (w231:T12)
            n100 = Bundle By Name(cluster=T22 {"Auto"=FALSE, "Accept"=FALSE, "Decline"=FALSE} ("Propose"), "Auto"=w230) -> (w229:T22)
            n101 = local write "Button States"(w231) -> ()
            n102 = local write "Execute"(w229) -> ()
          }
          frame #13 {
            n103 = Get Date/Time In Seconds() -> (seconds since 1Jan1904=w237:timestamp)
          }
        }
      }
      frame #1 {
      }
    }
    n104 = Unbundle By Name(w113) -> ("Exit Requested"=w114:bool)
  }
  n105 = while {
    shift-right: [w250] -> _
    shift-left: w12 -> [w252]
    shift-right: [w255] -> _
    shift-left: w29 -> [w259]
    shift-right: [w256] -> _
    shift-left: w3 -> [w258]
    tunnel: w4 -> [w251]
    tunnel: [w244] -> w55
    shift-right: [w246] -> _
    shift-left: w6 -> [w248]
    tunnel: w5 -> [w247]
    tunnel: w26 -> [w242]
    tunnel: w2 -> [w241]
    stop <- w244 stop-if-true
    # "Application\nEvents"
    n106 = Wait on Notification(notifier=w259, timeout in ms (-1)=200, error in (no error)=w258) -> (notifier out=w255:refnum<notifier>, notification=w254:T33, timed out?=w260:bool, error out=w257:errorcluster)  [unwired: 1 in]
    n107 = case shown="False" w260 {
      tunnel: w257 -> [w268 w315]
      tunnel: [w267 w315] -> w256
      tunnel: w254 -> [w273 _]
      tunnel: w252 -> [w270 w314]
      tunnel: w251 -> [w271 _]
      tunnel: [w269 w314] -> w250
      tunnel: [w266 _] -> w249
      tunnel: w248 -> [w265 w313]
      tunnel: w247 -> [w264 _]
      tunnel: [w263 w313] -> w246
      tunnel: w242 -> [w262 _]
      tunnel: w241 -> [w261 _]
      frame #0 {
        n108 = Unbundle By Name(w273) -> ("Command"=w272:T34)
        n109 = case shown="\"Control Enabled\"" w272 {
          tunnel: w271 -> [_ w290 w304 w312]
          tunnel: w270 -> [w276 w285 w299 w306]
          tunnel: [w276 w286 w300 w307] -> w269
          tunnel: w268 -> [w275 w287 w291 w309]
          tunnel: [w275 w282 w301 w308] -> w267
          tunnel: [_ w284 _ _] -> w266
          tunnel: w265 -> [w274 w280 w298 w305]
          tunnel: w264 -> [_ w279 w295 _]
          tunnel: [w274 w281 w297 w305] -> w263
          tunnel: w262 -> [_ _ _ _]
          tunnel: w261 -> [_ _ _ _]
          frame #0 {
          }
          frame #1 {
            w284 = TRUE ("Button States.Exit Requested")
            n110 = Bundle By Name(cluster=w290, "MM Control Events"=Mixed_Mode_Button_Events."Application.Stop", "Button States.Exit Requested"=w284) -> (w288:T35)
            n111 = Bundle By Name(cluster=w279, "MM GUI Update Type"=Mixed_Mode_GUI_Update_Type."Exit") -> (w278:T31)
            n112 = Send Notification(notification=w288, notifier=w285, error in (no error)=w287) -> (notifier out=w286:refnum<notifier>, error out=w283:errorcluster)
            n113 = Enqueue Element(queue=w280, element=w278, error in (no error)=w283) -> (queue out=w281:refnum<queue>, error out=w282:errorcluster)  [unwired: 1 in, 1 out]
          }
          frame #2 {
            n114 = Bundle By Name(cluster=w295, "MM GUI Update Type"=Mixed_Mode_GUI_Update_Type."Control.Enabled", "State"=TRUE) -> (w292:T31)
            n115 = Bundle By Name(cluster=w304, "MM Control Events"=Mixed_Mode_Button_Events."Control.Enabled") -> (w302:T35)
            n116 = Enqueue Element(queue=w298, element=w292, error in (no error)=w291) -> (queue out=w297:refnum<queue>, error out=w296:errorcluster)  [unwired: 1 in, 1 out]
            n117 = Send Notification(notification=w302, notifier=w299, error in (no error)=w296) -> (notifier out=w300:refnum<notifier>, error out=w301:errorcluster)
          }
          frame #3 {
            n118 = Bundle By Name(cluster=w312, "MM Control Events"=Mixed_Mode_Button_Events."Control.Disabled") -> (w310:T35)
            n119 = Send Notification(notification=w310, notifier=w306, error in (no error)=w309) -> (notifier out=w307:refnum<notifier>, error out=w308:errorcluster)
          }
        }
      }
      frame #1 {
      }
    }
    n120 = local read "Button States"() -> (w245:T12)
    n121 = Unbundle By Name(w245) -> ("Exit Requested"=w243:bool)
    n122 = Or(x=w243, y=w249) -> (x .or. y?=w244:bool)
  }
  n123 = while {
    shift-right: [w341] -> _
    shift-left: w12 -> [w327]
    shift-right: [w323] -> _
    shift-left: w43 -> [w340]
    tunnel: w4 -> [w337]
    shift-right: [w334] -> _
    shift-left: w29 -> [w335]
    tunnel: w28 -> [w333]
    tunnel: [w330] -> w56
    shift-right: [w328] -> _
    shift-left: w6 -> [w320]
    tunnel: w5 -> [w326]
    tunnel: w2 -> [w319]
    shift-right: [w317] -> _
    shift-left: w14 -> [w316]
    stop <- w330 stop-if-true
    # "Gui Events"
    n124 = local read "Button States"() -> (w338:T12)
    n125 = event shown="[11] \"Load File\": Mouse Down?" {
      selector: _ -> [_ _ _ _ _ _ _ _ _ _ _ _ _ _ _ _ _ _]
      dyn-events: _ -> [_ _ _ _ _ _ _ _ _ _ _ _ _ _ _ _ _ _]
      timeout: _ -> [_ _ _ _ _ _ _ _ _ _ _ _ _ _ _ _ _ w518]
      tunnel: [Mixed_Mode_Button_Events."Nop" ("MM Control Events") Mixed_Mode_Button_Events."Nop" ("MM Control Events") Mixed_Mode_Button_Events."Nop" ("MM Control Events") Mixed_Mode_Button_Events."Nop" ("MM Control Events") w403 Mixed_Mode_Button_Events."Propose.Accept" ("MM Control Events") Mixed_Mode_Button_Events."Propose.Decline" ("MM Control Events") Mixed_Mode_Button_Events."Execute.Start" ("MM Control Events") Mixed_Mode_Button_Events."Execute.Stop" ("MM Control Events") w446 Mixed_Mode_Button_Events."Nop" ("MM Control Events") Mixed_Mode_Button_Events."InputFile.Load" ("MM Control Events") Mixed_Mode_Button_Events."InputFile.Reset" ("MM Control Events") Mixed_Mode_Button_Events."InputFile.Run" ("MM Control Events") Mixed_Mode_Button_Events."Nop" ("MM Control Events") w503 Mixed_Mode_Button_Events."Nop" ("MM Control Events") Mixed_Mode_Button_Events."Nop" ("MM Control Events")] -> w342
      tunnel: w340 -> [w375 w383 w388 w394 w400 w414 w420 w426 w432 w437 w451 w464 w474 w482 w493 w506 w512 w521]
      tunnel: [w375 w383 w388 w394 w400 w414 w420 w426 w432 w436 w450 w463 w473 w482 w487 w506 w512 w520] -> w324
      tunnel: w338 -> [_ _ _ _ _ _ _ _ _ _ _ w466 _ w481 _ w504 _ _]
      tunnel: [_ _ _ _ _ _ _ _ _ _ _ w462 _ w480 _ w500 _ _] -> w336
      tunnel: [_ _ _ _ _ _ _ _ _ _ _ _ _ _ _ _ _ w526] -> w332
      tunnel: w335 -> [w374 w380 w387 w393 w402 w412 w418 w424 w430 w445 w456 w467 w475 w484 w494 w505 w511 w522]
      tunnel: [w374 w380 w387 w393 w402 w412 w418 w424 w430 w445 w456 w467 w475 w484 w494 w505 w511 w523] -> w334
      tunnel: w333 -> [_ _ _ _ _ _ _ _ _ _ _ _ _ _ _ _ _ w519]
      tunnel: [Mixed_Mode_GUI_Update_Type."Nop" ("MM GUI Update Type") Mixed_Mode_GUI_Update_Type."Nop" ("MM GUI Update Type") Mixed_Mode_GUI_Update_Type."Propose.Auto" ("MM GUI Update Type") Mixed_Mode_GUI_Update_Type."Execute.Auto" ("MM GUI Update Type") w401 Mixed_Mode_GUI_Update_Type."Nop" ("MM GUI Update Type") Mixed_Mode_GUI_Update_Type."Nop" ("MM GUI Update Type") Mixed_Mode_GUI_Update_Type."Nop" ("MM GUI Update Type") Mixed_Mode_GUI_Update_Type."Nop" ("MM GUI Update Type") Mixed_Mode_GUI_Update_Type."Nop" ("MM GUI Update Type") Mixed_Mode_GUI_Update_Type."Nop" ("MM GUI Update Type") Mixed_Mode_GUI_Update_Type."Input File Loaded" ("MM GUI Update Type") Mixed_Mode_GUI_Update_Type."Nop" ("MM GUI Update Type") Mixed_Mode_GUI_Update_Type."RunInputFile" ("MM GUI Update Type") Mixed_Mode_GUI_Update_Type."Nop" ("MM GUI Update Type") Mixed_Mode_GUI_Update_Type."NTCP Server" ("MM GUI Update Type") Mixed_Mode_GUI_Update_Type."Nop" ("MM GUI Update Type") Mixed_Mode_GUI_Update_Type."Nop" ("MM GUI Update Type")] -> w325
      tunnel: [_ _ w385 w392 _ _ _ _ _ _ _ w460 _ w478 _ w499 _ _] -> w321
      tunnel: w319 -> [w370 _ _ _ _ _ _ _ _ _ w454 _ _ _ _ _ _ _]
      tunnel: 200 -> [_ _ _ _ _ _ _ _ _ _ _ _ _ _ _ _ _ w518]
      tunnel: [w367 w379 w384 w390 w396 w409 w415 w421 w427 w433 w449 w459 w469 w477 w488 w498 w510 w517] -> w317
      tunnel: w316 -> [w367 w379 w384 w390 w396 w409 w415 w421 w427 w433 w449 w459 w469 w477 w489 w498 w510 w517]
      event #0 {
        n126 = event-data() -> ()  [unwired: 1 in, 7 out]
        n127 = local read "Mixed Mode Status"() -> (w377:T7)
        n128 = local read "Target Pattern"() -> (w378:T18)
        n129 = local read "Cartesian Type"() -> (w368:bool)
        n130 = call "Apply Target Pattern.vi"("Mixed Mode Status"=w377, "Target Pattern"=w378) -> ("Targets"=w369:T3[])  [unwired: 9 in]
        n131 = call "Current Target DAO.vi"("Combined"=w370, "Use Offsets"=w368, "Targets In"=w369, "DAO Actions"=DAO_Actions."Set") -> ()  [unwired: 6 in, 2 out]
        n132 = local write "Targets"(w369) -> ()
        n133 = event-data("Discard?"=TRUE) -> ()  [unwired: 1 in, 1 out]
      }
      event #1 {
        n134 = event-data() -> ()  [unwired: 1 in, 2 out]
      }
      event #2 {
        n135 = event-data() -> ("NewVal"=w385:bool)  [unwired: 1 in, 4 out]
      }
      event #3 {
        n136 = event-data() -> ("NewVal"=w392:bool)  [unwired: 1 in]
      }
      event #4 {
        n137 = event-data() -> ()  [unwired: 1 in, 7 out]
        n138 = call "Can Switch Control Types.vi"("DAO Actions"=DAO_Actions."Get") -> ("Can Switch Out"=w398:bool)  [unwired: 10 in]
        n139 = case shown="True" w398 {
          tunnel: [Mixed_Mode_Button_Events."Nop" ("MM Control Events") Mixed_Mode_Button_Events."ControlType.Changed" ("MM Control Events")] -> w403
          tunnel: [Mixed_Mode_GUI_Update_Type."Nop" ("MM GUI Update Type") Mixed_Mode_GUI_Update_Type."All Autos Off" ("MM GUI Update Type")] -> w401
          tunnel: [TRUE _] -> w397
          frame #0 {
          }
          frame #1 {
          }
        }
        n140 = event-data("Discard?"=w397) -> ()  [unwired: 4 in, 1 out]
      }
      event #5 {
        n141 = event-data() -> ()  [unwired: 1 in, 7 out]
        n142 = event-data("Discard?"=TRUE) -> ()  [unwired: 1 in, 1 out]
      }
      event #6 {
        n143 = event-data() -> ()  [unwired: 1 in, 7 out]
        n144 = event-data("Discard?"=TRUE) -> ()  [unwired: 1 in, 1 out]
      }
      event #7 {
        n145 = event-data() -> ()  [unwired: 1 in, 7 out]
        n146 = event-data("Discard?"=TRUE) -> ()  [unwired: 1 in, 1 out]
      }
      event #8 {
        n147 = event-data() -> ()  [unwired: 1 in, 7 out]
        n148 = event-data("Discard?"=TRUE) -> ()  [unwired: 1 in, 1 out]
      }
      event #9 {
        n149 = event-data() -> ()  [unwired: 1 in, 1 out]
        n150 = local read "Targets"() -> (w435:T3[])
        n151 = call "Fault List 2 Indicators.vi"("Use LBCB Selector"=FALSE) -> ("Forces"=w440:bool, "Displacement"=w441:bool)  [unwired: 7 in, 2 out]
        n152 = call "Clean Targets.vi"("Targets In"=w435, "error in"=w437) -> ("Problems"=w434:bool, "Targets Out"=w438:T3[], "error out"=w436:errorcluster)
        n153 = Compound Arithmetic op=OR(w441, w440, w434) -> (w442:bool)
        n154 = case shown="False" w442 {
          tunnel: [Mixed_Mode_Button_Events."Nop" ("MM Control Events") Mixed_Mode_Button_Events."TargetSet" ("MM Control Events")] -> w446
          frame #0 {
          }
          frame #1 {
          }
        }
        n155 = local write "Typo Problem"(w434) -> ()
        n156 = local write "Targets"(w438) -> ()
        n157 = event-data("Discard?"=TRUE) -> ()  [unwired: 1 in, 1 out]
      }
      event #10 {
        n158 = event-data() -> ("NewVal"=w452:T3[])  [unwired: 1 in]
        n159 = local read "Cartesian Type"() -> (w453:bool)
        n160 = call "Current Target DAO.vi"("Combined"=w454, "Use Offsets"=w453, "error in (no error)"=w451, "Targets In"=w452, "DAO Actions"=DAO_Actions."Set") -> ("error out"=w450:errorcluster)  [unwired: 5 in, 1 out]
      }
      event #11 {
        w460 = TRUE ("Input File Loaded")
        n161 = event-data() -> ()  [unwired: 1 in, 7 out]
        n162 = call "Input Files.vi"("error in (no error)"=w464) -> ("error out"=w463:errorcluster)  [unwired: 10 in]
        n163 = Bundle By Name(cluster=w466, "Input File Loaded"=w460) -> (w462:T12)
        n164 = event-data("Discard?"=TRUE) -> ()  [unwired: 1 in, 1 out]
      }
      event #12 {
        n165 = event-data() -> ()  [unwired: 1 in, 7 out]
        n166 = call "Input File Step Iterator.vi"("error in (no error)"=w474, "Input File Step Actions"=Input_File_Step_Actions."Reset") -> ("error out"=w473:errorcluster)  [unwired: 4 in, 3 out]
        n167 = event-data("Discard?"=TRUE) -> ()  [unwired: 1 in, 1 out]
      }
      event #13 {
        w478 = TRUE ("Input File Running")
        n168 = event-data() -> ()  [unwired: 1 in, 7 out]
        n169 = Bundle By Name(cluster=w481, "Input File Running"=w478) -> (w480:T12)
        n170 = event-data("Discard?"=TRUE) -> ()  [unwired: 1 in, 1 out]
      }
      event #14 {
        # "GUI is updated\nin the Application\nEvents loop"
        n171 = event-data() -> ("NewVal"=w491:bool)  [unwired: 1 in]
        n172 = Bundle By Name(cluster=T40 {"Cartesian Type"=FALSE, "Force Tag"="<None>"} ("Offset Out"), "Cartesian Type"=w491) -> (w492:T40)
        n173 = call "Offset Change Message DAO.vi"("error in (no error)"=w493, "Offset In"=w492, "DAO Actions"=DAO_Actions."Set") -> ("error out"=w486:errorcluster)  [unwired: 6 in, 2 out]
        n174 = Send Notification(notification=w491, notifier=w489, error in (no error)=w486) -> (notifier out=w488:refnum<notifier>, error out=w487:errorcluster)
      }
      event #15 {
        n175 = event-data() -> ("NewVal"=w499:bool)  [unwired: 1 in]
        n176 = Bundle By Name(cluster=w504, "NTCP Server  On"=w499) -> (w500:T12)
        n177 = Select(t=Mixed_Mode_Button_Events."NCTP.ConnectToServer" ("MM Control Events"), s=w499, f=Mixed_Mode_Button_Events."NTCP.DisconnectFromServer") -> (s? t:f=w503:T36)
      }
      event #16 {
        n178 = event-data() -> ("NewVal"=w513:cluster{"Displacement":T15, "Force":T15})  [unwired: 1 in]
        n179 = call "Persistant Ramp Time DAO.vi"("Ramp Time Actions"=Persistant_DAO_Actions."Set", "Ramp Time In"=w513) -> ()  [unwired: 2 in, 12 out]
      }
      event #17 {
        # "GUI is updated\nin the Application\nEvents loop"
        n180 = event-data() -> ("NewVal"=w526:bool)  [unwired: 1 in]
        n181 = Bundle By Name(cluster=w519, "Command"=MM_Widget_Parameter_Changes."Stop All") -> (w525:T33)
        n182 = Send Notification(notification=w525, notifier=w522, error in (no error)=w521) -> (notifier out=w523:refnum<notifier>, error out=w520:errorcluster)
      }
    }
    n183 = local read "Button States"() -> (w331:T12)
    n184 = Unbundle By Name(w331) -> ("Exit Requested"=w329:bool)
    n185 = Or(x=w329, y=w332) -> (x .or. y?=w330:bool)
    n186 = case shown="\"All Autos Off\"" w325 {
      selector: w325 -> [_ w349 _]
      tunnel: w320 -> [w344 w352 w356]
      tunnel: [w344 w351 w354] -> w328
      tunnel: w326 -> [_ w350 _]
      tunnel: w324 -> [w343 w347 w355]
      tunnel: [w343 w346 w353] -> w322
      tunnel: w321 -> [_ w345 _]
      frame #0 {
      }
      frame #1 {
        n187 = Bundle By Name(cluster=w350, "MM GUI Update Type"=w349, "State"=w345) -> (w348:T31)
        n188 = Enqueue Element(queue=w352, element=w348, error in (no error)=w347) -> (queue out=w351:refnum<queue>, error out=w346:errorcluster)  [unwired: 1 in, 1 out]
      }
      frame #2 {
        n189 = call "Autos Off.vi"("error in"=w355, "queue in"=w356) -> ("error out"=w353:errorcluster, "queue out"=w354:refnum<queue>)  [unwired: 2 in]
      }
    }
    n190 = case shown="\"Propose.Accept\", Default" w342 {
      selector: w342 -> [w358 _]
      tunnel: w327 -> [w364 w366]
      tunnel: [w363 w366] -> w341
      tunnel: w324 -> [w362 w365]
      tunnel: [w361 w365] -> w339
      tunnel: w337 -> [w360 _]
      tunnel: w336 -> [w357 _]
      frame #0 {
        n191 = Bundle By Name(cluster=w360, "MM Control Events"=w358, "Button States"=w357) -> (w359:T35)
        n192 = Send Notification(notification=w359, notifier=w364, error in (no error)=w362) -> (notifier out=w363:refnum<notifier>, error out=w361:errorcluster)
      }
      frame #1 {
      }
    }
    n193 = call <vilib>:"Merge Errors.vi"("error in 3 (no error)"=w339, "error in 2 (no error)"=w322) -> ("error out"=w323:errorcluster)  [unwired: 5 in]
  }
  n194 = while {
    shift-right: [w528] -> _
    shift-left: w12 -> [w531]
    shift-right: [w527] -> _
    shift-left: w10 -> [w537]
    tunnel: w9 -> [w536]
    shift-right: [w532] -> _
    shift-left: w6 -> [w533]
    tunnel: w5 -> [w534]
    tunnel: w4 -> [w530]
    stop <- w540 stop-if-true
    n195 = Wait on Notification(notifier=w536, timeout in ms (-1)=2000, error in (no error)=w537) -> (timed out?=w535:bool, error out=w529:errorcluster)  [unwired: 1 in, 2 out]
    n196 = case shown="False" w535 {
      tunnel: w534 -> [w548 _]
      tunnel: w533 -> [w547 w571]
      tunnel: [w546 w571] -> w532
      tunnel: w531 -> [w545 w569]
      tunnel: w530 -> [w544 _]
      tunnel: w529 -> [w543 w570]
      tunnel: [w542 w569] -> w528
      tunnel: [w541 w570] -> w527
      frame #0 {
        n197 = call "NTCP Server Change Message DAO.vi"("DAO Actions"=DAO_Actions."Get") -> ("NTCP Change Out"=w549:bool)  [unwired: 8 in, 2 out]
        n198 = case shown="False" w549 {
          selector: w549 -> [w560 _]
          tunnel: w548 -> [w565 _]
          tunnel: w547 -> [w564 w568]
          tunnel: [w563 w568] -> w546
          tunnel: w545 -> [w559 w567]
          tunnel: w544 -> [w558 _]
          tunnel: w543 -> [w557 w566]
          tunnel: [w556 w567] -> w542
          tunnel: [w551 w566] -> w541
          frame #0 {
            n199 = Bundle By Name(cluster=w558, "MM Control Events"=Mixed_Mode_Button_Events."NTCP.DisconnectFromServer") -> (w555:T35)
            n200 = Bundle By Name(cluster=w565, "MM GUI Update Type"=Mixed_Mode_GUI_Update_Type."NTCP Server", "State"=w560) -> (w562:T31)
            n201 = Send Notification(notification=w555, notifier=w559, error in (no error)=w557) -> (notifier out=w556:refnum<notifier>, error out=w552:errorcluster)
            n202 = Enqueue Element At Opposite End(queue=w564, element=w562, error in (no error)=w557) -> (queue out=w563:refnum<queue>, error out=w553:errorcluster)  [unwired: 1 in, 1 out]
            n203 = call <vilib>:"Merge Errors.vi"("error in 2 (no error)"=w552, "error in 1 (no error)"=w553) -> ("error out"=w551:errorcluster)  [unwired: 5 in]
          }
          frame #1 {
          }
        }
      }
      frame #1 {
      }
    }
    n204 = local read "Button States"() -> (w539:T12)
    n205 = Unbundle By Name(w539) -> ("Exit Requested"=w540:bool)
  }
  n206 = while {
    shift-right: [w578] -> _
    shift-left: w14 -> [w583]
    shift-right: [w579] -> _
    shift-left: w13 -> [w582]
    shift-right: [w575] -> _
    shift-left: w12 -> [w577]
    shift-right: [w574] -> _
    shift-left: w6 -> [w576]
    tunnel: w4 -> [w573]
    tunnel: w2 -> [w572]
    stop <- w586 stop-if-true
    # "Offset Change Loop"
    n207 = Wait on Notification(notifier=w583, timeout in ms (-1)=2000, error in (no error)=w582) -> (notifier out=w578:refnum<notifier>, timed out?=w581:bool, error out=w580:errorcluster)  [unwired: 1 in, 1 out]
    n208 = case shown="False" w581 {
      tunnel: w580 -> [w604 w610]
      tunnel: [w603 w610] -> w579
      tunnel: w577 -> [w602 w611]
      tunnel: w576 -> [w601 w609]
      tunnel: [w600 w611] -> w575
      tunnel: [w599 w609] -> w574
      tunnel: w573 -> [w598 _]
      tunnel: w572 -> [w597 _]
      frame #0 {
        w588 = T29 TRUE ("Use Offsets")
        n209 = call "Offset Change Message DAO.vi"("DAO Actions"=DAO_Actions."Get") -> ("Offset Out"=w605:T40)  [unwired: 8 in, 2 out]
        n210 = Unbundle By Name(w605) -> ("Cartesian Type"=w596:bool, "Force Tag"=w589:string)
        n211 = local write "Force Tag"(w589) -> ()
        n212 = local read "Targets"() -> (w595:T3[])
        n213 = Select(t=enum16{" +", " - "}." - " ("Direction"), s=w596, f=enum16{" +", " - "}." +") -> (s? t:f=w590:enum16{" +", " - "})
        n214 = local write "Cartesian Type"(w596) -> ()
        n215 = Bundle By Name(cluster=w598, "MM Control Events"=Mixed_Mode_Button_Events."CartesianType.Changed") -> (w608:T35)
        n216 = call "Local2Global Target Values.vi"("Tag"="<None>" ("Current Tag"), "Direction"=w590, "Use Offsets"=w588, "Combined"=w597, "AreCommands"=w588, "Target  Inputs"=w595) -> ("Target  Outputs"=w594:T3[])  [unwired: 5 in]
        n217 = call "Autos Off.vi"("error in"=w604, "Cartesian Type"=w596, "Targets"=w594, "queue in"=w601) -> ("error out"=w593:errorcluster, "queue out"=w599:refnum<queue>)
        n218 = Send Notification(notification=w608, notifier=w602, error in (no error)=w593) -> (notifier out=w600:refnum<notifier>, error out=w603:errorcluster)
      }
      frame #1 {
      }
    }
    n219 = local read "Button States"() -> (w585:T12)
    n220 = Unbundle By Name(w585) -> ("Exit Requested"=w586:bool)
  }
  n221 = Obtain Notifier(name (unnamed)="Mixed Mode Statuses", notification data type=T7 {"LBCB Target"=[], "MixedModeStates"=enum."Init", "LBCB Convergence"=[], "LBCB Measurements"=[]} ("Mixed Mode Status"), error in (no error)=w43) -> (notifier out=w48:refnum<notifier>, error out=w47:errorcluster)  [unwired: 1 in, 1 out]
  n222 = Obtain Queue(name (unnamed)="Mixed Mode State", element data type=Mixed_Mode_States."Init" ("f"), error in (no error)=w43) -> (queue out=w44:refnum<queue>, error out=w33:errorcluster)  [unwired: 2 in, 1 out]
  n223 = Obtain Queue(name (unnamed)="MCL States", element data type=MCL_States."MCL Idle" ("MCL States"), error in (no error)=w33) -> (queue out=w31:refnum<queue>, error out=w20:errorcluster)  [unwired: 2 in, 1 out]
  n224 = Obtain Queue(name (unnamed)="Proxy Mixed Mode State", element data type=w17, error in (no error)=w20) -> (queue out=w18:refnum<queue>, error out=w19:errorcluster)  [unwired: 2 in, 1 out]
  n225 = while {
    tunnel: [w631] -> w35
    shift-right: [w629] -> _
    shift-left: Input_File_States."InputFile.Idle" ("Input File States") -> [w630]
    shift-right: [w620] -> _
    shift-left: w12 -> [w621]
    shift-right: [w625] -> _
    shift-left: w10 -> [w626]
    shift-right: [w624] -> _
    shift-left: w6 -> [w627]
    shift-right: [w616] -> _
    shift-left: w31 -> [w617]
    shift-right: [w618] -> _
    shift-left: w27 -> [w619]
    tunnel: w5 -> [w622]
    tunnel: w2 -> [w612]
    stop <- w631 stop-if-true
    # "Input File States"
    n226 = local read "Mixed Mode Control Tabs"() -> (w615:enum32{"Manual", "Input File", "NTCP"})
    n227 = local read "Button States"() -> (w632:T12)
    n228 = Unbundle By Name(w632) -> ("Auto-Accept Enabled"=w614:bool, "Auto-Start Enabled"=w613:bool, "Input File Loaded"=w628:bool, "Exit Requested"=w631:bool)
    n229 = case shown="\"Input File\"" w615 {
      tunnel: w630 -> [_ w657]
      tunnel: [Input_File_States."InputFile.Idle" ("Input File States") w656] -> w629
      tunnel: w628 -> [_ w655]
      tunnel: w627 -> [w636 w654]
      tunnel: w626 -> [w635 w653]
      tunnel: [w635 w652] -> w625
      tunnel: [w636 w651] -> w624
      tunnel: 200 ("timeout in ms (-1)") -> [_ w643]
      tunnel: w622 -> [_ w650]
      tunnel: w621 -> [w637 w649]
      tunnel: [w637 w648] -> w620
      tunnel: w619 -> [w633 w647]
      tunnel: [w633 w646] -> w618
      tunnel: w617 -> [w634 w645]
      tunnel: [w634 w644] -> w616
      tunnel: w614 -> [_ w642]
      tunnel: w613 -> [_ w641]
      tunnel: w612 -> [_ w640]
      frame #0 {
        n230 = Wait Until Next ms Multiple(millisecond multiple=u32 200) -> ()  [unwired: 1 out]
      }
      frame #1 {
        n231 = case shown="\"InputFile.StopRunning\"" w657 {
          selector: w657 -> [w666 w669 _ _ w757 w778 w806 w828 _]
          tunnel: [w668 w670 w724 w747 w758 w779 w805 w830 Input_File_States."InputFile.Idle" ("Input File States")] -> w656
          tunnel: w655 -> [w667 _ _ _ _ _ _ _ _]
          tunnel: w654 -> [w663 w676 w723 w752 w764 w784 w812 w832 w849]
          tunnel: w653 -> [w664 w681 w717 w741 w763 w783 w802 w825 w838]
          tunnel: [w664 w671 w716 w736 w762 w774 w810 w824 w840] -> w652
          tunnel: [w663 w672 w723 w734 w761 w781 w812 w832 w841] -> w651
          tunnel: w650 -> [_ w675 _ w732 _ _ _ _ w852]
          tunnel: w649 -> [w660 w682 w720 w749 w765 w785 w817 w826 w847]
          tunnel: [w660 w680 w719 w748 w760 w782 w816 w826 w847] -> w648
          tunnel: w647 -> [w662 w678 w721 w743 w756 w773 w818 w827 w845]
          tunnel: [w662 w678 w721 w743 w756 w772 w815 w827 w845] -> w646
          tunnel: w645 -> [w661 w679 w722 w744 w755 w776 w814 w834 w846]
          tunnel: [w661 w679 w722 w744 w755 w776 w813 w833 w846] -> w644
          tunnel: w643 -> [_ w673 w718 w742 w754 w777 w807 w829 _]
          tunnel: w642 -> [_ _ _ _ w753 _ _ _ _]
          tunnel: w641 -> [_ _ _ _ _ w771 _ _ _]
          tunnel: w640 -> [_ _ _ _ _ w770 _ _ _]
          frame #0 {
            n232 = call "Can Switch Control Types.vi"("Can Switch In"=TRUE, "DAO Actions"=DAO_Actions."Set") -> ()  [unwired: 9 in, 1 out]
            n233 = Select(t=Input_File_States."InputFile.WaitForRunning" ("Input File States"), s=w667, f=w666) -> (s? t:f=w668:T20)
          }
          frame #1 {
            n234 = call "Input File Run or Stop.vi"("timeout"=w673, "error in (no error)"=w681, "MM Button Events In"=w682) -> ("error out"=w674:errorcluster, "Running"=w677:T49, "Button Events Out"=w680:refnum<notifier>)  [unwired: 6 in]
            n235 = case shown="\"Run\"" w677 {
              tunnel: w676 -> [w685 w690 w702]
              tunnel: w675 -> [_ w695 w707]
              tunnel: w674 -> [w684 w691 w703]
              tunnel: w673 -> [_ w689 w701]
              tunnel: [w685 w688 w700] -> w672
              tunnel: [w684 w687 w699] -> w671
              tunnel: [w683 Input_File_States."InputFile.WaitForRunning" ("Input File States") Input_File_States."InputFile.StepsAvailable" ("Input File States")] -> w670
              tunnel: w669 -> [w683 _ _]
              frame #0 {
              }
              frame #1 {
                n236 = Bundle By Name(cluster=w695, "MM GUI Update Type"=Mixed_Mode_GUI_Update_Type."RunInputFile", "State"=FALSE) -> (w694:T31)
                n237 = Enqueue Element(queue=w690, element=w694, timeout in ms (-1)=w689, error in (no error)=w691) -> (queue out=w688:refnum<queue>, error out=w687:errorcluster)  [unwired: 1 out]
              }
              frame #2 {
                n238 = Bundle By Name(cluster=w707, "MM GUI Update Type"=Mixed_Mode_GUI_Update_Type."RunInputFile", "State"=TRUE) -> (w706:T31)
                n239 = call "Can Switch Control Types.vi"("Can Switch In"=FALSE, "DAO Actions"=DAO_Actions."Set") -> ()  [unwired: 9 in, 1 out]
                n240 = Enqueue Element(queue=w702, element=w706, timeout in ms (-1)=w701, error in (no error)=w703) -> (queue out=w700:refnum<queue>, error out=w699:errorcluster)  [unwired: 1 out]
              }
            }
          }
          frame #2 {
            w711 = Input_File_States."InputFile.StopRunning" ("t")
            n241 = call "Input File Run or Stop.vi"("timeout"=w718, "error in (no error)"=w717, "MM Button Events In"=w720) -> ("error out"=w716:errorcluster, "Running"=w709:T49, "Button Events Out"=w719:refnum<notifier>)  [unwired: 6 in]
            n242 = Not Equal?(x=w709, y=Run_Or_Stop_Result."Stop") -> (x != y?=w710:bool)
            n243 = call "Input File Step Iterator.vi"("Input File Step Actions"=Input_File_Step_Actions."Next Step") -> ("End of Input File"=w714:bool)  [unwired: 5 in, 3 out]
            n244 = Select(t=w711, s=w714, f=Input_File_States."InputFile.LoadStep") -> (s? t:f=w713:T20)
            n245 = Select(t=w713, s=w710, f=w711) -> (s? t:f=w724:T20)
          }
          frame #3 {
            n246 = call "Input File Step Iterator.vi"("Input File Step Actions"=Input_File_Step_Actions."Get Step") -> ("Next Step"=w750:T50)  [unwired: 5 in, 3 out]
            n247 = Unbundle By Name(w750) -> ("Targets"=w727:T3[], "Step Number"=w730:u32)
            n248 = local read "Cartesian Type"() -> (w726:bool)
            n249 = call "Input File Run or Stop.vi"("timeout"=w742, "error in (no error)"=w741, "MM Button Events In"=w749) -> ("Running"=w739:T49, "Button Events Out"=w748:refnum<notifier>)  [unwired: 6 in, 1 out]
            n250 = Bundle By Name(cluster=w732, "MM GUI Update Type"=Mixed_Mode_GUI_Update_Type."Targets", "Targets"=w727, "State"=w726) -> (w728:T31)
            n251 = call "Steps DAO.vi"("Step In"=w730, "Steps Actions"=T38."Set Step") -> ("Step String Out"=w729:string)  [unwired: 7 in, 2 out]
            n252 = Bundle By Name(cluster=w732, "MM GUI Update Type"=Mixed_Mode_GUI_Update_Type."TestStats", "Step"=w729) -> (w733:T31)
            n253 = Enqueue Element(queue=w752, element=w728, timeout in ms (-1)=w742, error in (no error)=w741) -> (queue out=w735:refnum<queue>, error out=w736:errorcluster)  [unwired: 1 out]
            n254 = Equal?(x=w739, y=Run_Or_Stop_Result."Stop") -> (x = y?=w738:bool)
            n255 = Enqueue Element(queue=w735, element=w733, error in (no error)=w736) -> (queue out=w734:refnum<queue>)  [unwired: 1 in, 2 out]
            n256 = Select(t=Input_File_States."InputFile.StopRunning" ("f"), s=w738, f=Input_File_States."InputFile.WaitForAccept") -> (s? t:f=w747:T20)
          }
          frame #4 {
            n257 = call "Accept Or Decline.vi"("timeout"=w754, "error in (no error)"=w763, "AutoAccept"=w753, "MM Gui Updates In"=w764, "MM Button Events In"=w765) -> ("error out"=w762:errorcluster, "Accepted or Declined"=w759:T51, "MM Gui Updates Out"=w761:refnum<queue>, "Button Events Out"=w760:refnum<notifier>)  [unwired: 3 in]
            n258 = case shown="\"Accepted\"" w759 {
              tunnel: [w766 Input_File_States."InputFile.WaitForStart" ("f") Input_File_States."InputFile.StopRunning" ("f") Input_File_States."InputFile.StopRunning" ("f")] -> w758
              tunnel: w757 -> [w766 _ _ _]
              frame #0 {
              }
              frame #1 {
              }
              frame #2 {
              }
              frame #3 {
              }
            }
          }
          frame #5 {
            n259 = call "Start Or Stop.vi"("timeout"=w777, "error in (no error)"=w783, "AutoStart"=w771, "MM Gui Updates In"=w784, "MM Button Events In"=w785) -> ("error out"=w775:errorcluster, "Start or Stop"=w780:T51, "MM Gui Updates Out"=w781:refnum<queue>, "Button Events Out"=w782:refnum<notifier>)  [unwired: 3 in]
            n260 = case shown="\"Accepted\"" w780 {
              tunnel: [w788 Input_File_States."InputFile.WaitForMclRamp" ("f") Input_File_States."InputFile.StopRunning" ("f") Input_File_States."InputFile.StopRunning" ("f")] -> w779
              tunnel: w778 -> [w788 _ _ _]
              tunnel: w775 -> [w786 w794 w796 w799]
              tunnel: [w786 w793 w796 w799] -> w774
              tunnel: w773 -> [w787 w792 w797 w800]
              tunnel: [w787 w791 w797 w800] -> w772
              tunnel: w770 -> [_ w789 _ _]
              frame #0 {
              }
              frame #1 {
                n261 = local read "Ramp Times"() -> (w790:cluster{"Displacement":T15, "Force":T15})
                n262 = call "Send Mixed Mode Command.vi"("MCL Command In"=w792, "Ramp Times"=w790, "error in"=w794, "Combined"=w789) -> ("MCL Command Out"=w791:refnum<queue>, "error out"=w793:errorcluster)  [unwired: 1 in]
              }
              frame #2 {
              }
              frame #3 {
              }
            }
          }
          frame #6 {
            n263 = call "Done Or Abort.vi"("error in (no error)"=w802, "timeout"=w807, "MCL State In"=w814) -> ("error out"=w809:errorcluster, "MCL State"=w811:T52, "MCL State Out"=w813:refnum<queue>)  [unwired: 1 in]
            n264 = case shown="\"Abort\"" w811 {
              tunnel: [Input_File_States."InputFile.StepsAvailable" ("f") Input_File_States."InputFile.StopRunning" ("f") w823] -> w804
              tunnel: w806 -> [_ _ w823]
              frame #0 {
              }
              frame #1 {
              }
              frame #2 {
              }
            }
            n265 = call "Monitor for Stop.vi"("timeout"=w807, "error in (no error)"=w802, "Mixed Mode Commands In"=w818, "MM Button Events In"=w817) -> ("error out"=w808:errorcluster, "Mixed Mode Commands Out"=w815:refnum<queue>, "Stop Requests"=w803:T53, "Button Events Out"=w816:refnum<notifier>)  [unwired: 4 in]
            n266 = case shown="\"Stop Requested\", Default" w803 {
              tunnel: [w819 Input_File_States."InputFile.StopRunning" ("f")] -> w805
              tunnel: w804 -> [w819 _]
              frame #0 {
              }
              frame #1 {
              }
            }
            n267 = call <vilib>:"Merge Errors.vi"("error in 3 (no error)"=w809, "error in 1 (no error)"=w808) -> ("error out"=w810:errorcluster)  [unwired: 5 in]
          }
          frame #7 {
            n268 = call "MCL Ramping.vi"("error in (no error)"=w825, "timeout"=w829, "MCL State In"=w834) -> ("error out"=w824:errorcluster, "Is Ramping?"=w831:bool, "MCL State Out"=w833:refnum<queue>)  [unwired: 1 in]
            n269 = case shown="True" w831 {
              tunnel: [w835 Input_File_States."InputFile.WaitForMclDone" ("Input File States")] -> w830
              tunnel: w828 -> [w835 _]
              frame #0 {
              }
              frame #1 {
              }
            }
          }
          frame #8 {
            n270 = Bundle By Name(cluster=w852, "MM GUI Update Type"=Mixed_Mode_GUI_Update_Type."RunInputFile", "State"=FALSE) -> (w848:T31)
            n271 = call "Input File Step Iterator.vi"("error in (no error)"=w838, "Input File Step Actions"=Input_File_Step_Actions."Backup") -> ("error out"=w837:errorcluster)  [unwired: 4 in, 3 out]
            n272 = Enqueue Element(queue=w849, element=w848, error in (no error)=w837) -> (queue out=w843:refnum<queue>, error out=w842:errorcluster)  [unwired: 1 in, 1 out]
            n273 = call "Autos Off.vi"("error in"=w842, "queue in"=w843) -> ("error out"=w840:errorcluster, "queue out"=w841:refnum<queue>)  [unwired: 2 in]
          }
        }
      }
    }
    "Input File States" <- w629
  }
  n274 = while {
    shift-right: [w869] -> _
    shift-left: w12 -> [w871]
    shift-right: [w867] -> _
    shift-left: w33 -> [w870]
    shift-right: [w866] -> _
    shift-left: w6 -> [w868]
    shift-right: [w863] -> _
    shift-left: w31 -> [w865]
    shift-right: [w859] -> _
    shift-left: Manual_States."Manual.Idle" ("Manual States") -> [w872]
    shift-right: [w861] -> _
    shift-left: w27 -> [w862]
    tunnel: [w860] -> w36
    tunnel: w5 -> [w856]
    tunnel: w2 -> [w855]
    shift-right: [w854] -> _
    shift-left: FALSE -> [w853]
    stop <- w860 stop-if-true
    # "Manual States"
    n275 = local read "Mixed Mode Control Tabs"() -> (w858:enum32{"Manual", "Input File", "NTCP"})
    n276 = local read "Button States"() -> (w873:T12)
    n277 = Unbundle By Name(w873) -> ("Auto-Start Enabled"=w857:bool, "Exit Requested"=w860:bool)
    n278 = case shown="\"Manual\"" w858 {
      tunnel: [w888 Manual_States."Manual.Idle" ("Manual States")] -> w859
      tunnel: w872 -> [w891 _]
      tunnel: w871 -> [w890 w1039]
      tunnel: w870 -> [w889 w1038]
      tunnel: [w887 w1039] -> w869
      tunnel: w868 -> [w886 w1037]
      tunnel: [w885 w1038] -> w867
      tunnel: [w884 w1037] -> w866
      tunnel: w865 -> [w883 w1036]
      tunnel: 200 ("timeout in ms (-1)") -> [w882 _]
      tunnel: [w881 w1036] -> w863
      tunnel: w862 -> [w880 w1035]
      tunnel: [w879 w1035] -> w861
      tunnel: w857 -> [w878 _]
      tunnel: w856 -> [w877 _]
      tunnel: w855 -> [w876 _]
      tunnel: [w875 w1034] -> w854
      tunnel: w853 -> [w874 w1034]
      frame #0 {
        n279 = case shown="\"Manual.WaitForStart\"" w891 {
          selector: w891 -> [_ _ _ w996 w1017 _]
          tunnel: w890 -> [w906 w946 w986 w998 w1012 w1033]
          tunnel: w889 -> [w905 w944 w984 w999 w1013 w1028]
          tunnel: [w903 w941 Manual_States."Manual.WaitForMclDone" ("Manual States") w1002 w1018 Manual_States."Manual.Idle" ("Manual States")] -> w888
          tunnel: [w902 w943 w986 w997 w1012 w1033] -> w887
          tunnel: w886 -> [w898 w945 w985 w1004 w1020 w1029]
          tunnel: [w899 w937 w988 w994 w1015 w1026] -> w885
          tunnel: [w898 w931 w985 w1004 w1020 w1027] -> w884
          tunnel: w883 -> [w897 w940 w990 w1007 w1022 w1032]
          tunnel: w882 -> [w900 w935 _ w995 w1016 _]
          tunnel: [w897 w940 w990 w1006 w1021 w1032] -> w881
          tunnel: w880 -> [w896 w939 w989 w1001 w1014 w1030]
          tunnel: [w896 w936 w987 w1000 w1014 w1030] -> w879
          tunnel: w878 -> [_ w934 _ _ _ _]
          tunnel: w877 -> [_ w933 _ _ _ _]
          tunnel: w876 -> [_ w930 _ _ _ _]
          tunnel: [w893 w929 w980 w992 w1011 w1025] -> w875
          tunnel: w874 -> [w892 w929 w980 w992 w1011 w1025]
          frame #0 {
            n280 = call "Can Switch Control Types.vi"("Can Switch In"=TRUE, "DAO Actions"=DAO_Actions."Set") -> ()  [unwired: 9 in, 1 out]
            n281 = Wait on Notification(notifier=w906, timeout in ms (-1)=w900, error in (no error)=w905) -> (notifier out=w902:refnum<notifier>, notification=w901:T35, timed out?=w904:bool, error out=w899:errorcluster)  [unwired: 1 in]
            n282 = case shown="False" w904 {
              tunnel: [w909 Manual_States."Manual.Idle" ("Manual States")] -> w903
              tunnel: w901 -> [w911 _]
              tunnel: [w908 w927] -> w893
              tunnel: w892 -> [w907 w927]
              frame #0 {
                n283 = Unbundle By Name(w911) -> ("MM Control Events"=w910:T36)
                n284 = case shown="\"TargetSet\"" w910 {
                  tunnel: [Manual_States."Manual.WaitForStart" ("t") Manual_States."Manual.Idle" ("Manual States") w918 w920 Manual_States."Manual.Idle" ("t")] -> w909
                  tunnel: [w912 w914 w917 TRUE FALSE] -> w908
                  tunnel: w907 -> [w912 w914 w917 w921 _]
                  frame #0 {
                  }
                  frame #1 {
                  }
                  frame #2 {
                    n285 = Select(t=Manual_States."Manual.Idle", s=w917, f=Manual_States."Manual.InitialPosition") -> (s? t:f=w918:T19)
                  }
                  frame #3 {
                    n286 = Select(t=Manual_States."Manual.Idle", s=w921, f=Manual_States."Manual.InitialPosition") -> (s? t:f=w920:T19)
                  }
                  frame #4 {
                  }
                }
              }
              frame #1 {
              }
            }
          }
          frame #1 {
            n287 = call "Start Or Stop.vi"("timeout"=w935, "error in (no error)"=w944, "AutoStart"=w934, "MM Gui Updates In"=w945, "MM Button Events In"=w946) -> ("error out"=w938:errorcluster, "Start or Stop"=w942:T51, "MM Gui Updates Out"=w932:refnum<queue>, "Button Events Out"=w943:refnum<notifier>)  [unwired: 3 in]
            n288 = case shown="\"Accepted\"" w942 {
              tunnel: [Manual_States."Manual.WaitForStart" ("Manual States") Manual_States."Manual.WaitForMclRamp" ("Manual States") Manual_States."Manual.Abort" ("Manual States") Manual_States."Manual.Abort" ("Manual States")] -> w941
              tunnel: w939 -> [w948 w970 w974 w978]
              tunnel: w938 -> [w949 w968 w973 w977]
              tunnel: [w949 w952 w973 w977] -> w937
              tunnel: [w948 w967 w974 w978] -> w936
              tunnel: w933 -> [_ w956 _ _]
              tunnel: w932 -> [w947 w955 w972 w976]
              tunnel: [w947 w954 w972 w976] -> w931
              tunnel: w930 -> [_ w951 _ _]
              frame #0 {
              }
              frame #1 {
                n289 = local read "Ramp Times"() -> (w969:cluster{"Displacement":T15, "Force":T15})
                n290 = call "Can Switch Control Types.vi"("Can Switch In"=FALSE, "DAO Actions"=DAO_Actions."Set") -> ()  [unwired: 9 in, 1 out]
                n291 = call "Send Mixed Mode Command.vi"("MCL Command In"=w970, "Ramp Times"=w969, "error in"=w968, "Combined"=w951) -> ("MCL Command Out"=w967:refnum<queue>, "error out"=w953:errorcluster)  [unwired: 1 in]
                n292 = call "Steps DAO.vi"("Steps Actions"=T38."Get Step String") -> ("Steps Out"=w963:T54)  [unwired: 8 in, 2 out]
                n293 = Unbundle By Name(w963) -> ("Correction Step"=w960:i32)
                n294 = Increment(x=w960) -> (x+1=w961:i32)
                n295 = call "Steps DAO.vi"("Step In"=w961, "Steps Actions"=T38."Set Correction Step") -> ("Step String Out"=w957:string)  [unwired: 7 in, 2 out]
                n296 = Bundle By Name(cluster=w956, "MM GUI Update Type"=Mixed_Mode_GUI_Update_Type."TestStats", "Step"=w957) -> (w958:T31)
                n297 = Enqueue Element(queue=w955, element=w958, error in (no error)=w953) -> (queue out=w954:refnum<queue>, error out=w952:errorcluster)  [unwired: 1 in, 1 out]
              }
              frame #2 {
              }
              frame #3 {
              }
            }
          }
          frame #2 {
            n298 = local read "Ramp Times"() -> (w981:cluster{"Displacement":T15, "Force":T15})
            n299 = call "Can Switch Control Types.vi"("Can Switch In"=FALSE, "DAO Actions"=DAO_Actions."Set") -> ()  [unwired: 9 in, 1 out]
            n300 = call "Send Initial Position Command.vi"("MCL Command In"=w989, "Ramp Times"=w981, "error in"=w984) -> ("MCL Command Out"=w987:refnum<queue>, "error out"=w988:errorcluster)  [unwired: 2 in]
          }
          frame #3 {
            n301 = call "Done Or Abort.vi"("timeout"=w995, "MCL State In"=w1007) -> ("error out"=w1005:errorcluster, "MCL State"=w1003:T52, "MCL State Out"=w1006:refnum<queue>)  [unwired: 2 in]
            n302 = call "Monitor for Stop.vi"("timeout"=w995, "error in (no error)"=w999, "Mixed Mode Commands In"=w1001, "MM Button Events In"=w998) -> ("error out"=w993:errorcluster, "Mixed Mode Commands Out"=w1000:refnum<queue>, "Button Events Out"=w997:refnum<notifier>)  [unwired: 4 in, 1 out]
            n303 = case shown="\"Abort\"" w1003 {
              tunnel: [Manual_States."Manual.Idle" ("Manual States") Manual_States."Manual.Abort" ("Manual States") w1010] -> w1002
              tunnel: w996 -> [_ _ w1010]
              frame #0 {
              }
              frame #1 {
              }
              frame #2 {
              }
            }
            n304 = call <vilib>:"Merge Errors.vi"("error in 3 (no error)"=w1005, "error in 1 (no error)"=w993) -> ("error out"=w994:errorcluster)  [unwired: 5 in]
          }
          frame #4 {
            n305 = call "MCL Ramping.vi"("error in (no error)"=w1013, "timeout"=w1016, "MCL State In"=w1022) -> ("error out"=w1015:errorcluster, "Is Ramping?"=w1019:bool, "MCL State Out"=w1021:refnum<queue>)  [unwired: 1 in]
            n306 = case shown="True" w1019 {
              tunnel: [w1023 Manual_States."Manual.WaitForMclDone" ("Manual States")] -> w1018
              tunnel: w1017 -> [w1023 _]
              frame #0 {
              }
              frame #1 {
              }
            }
          }
          frame #5 {
            n307 = call "Autos Off.vi"("error in"=w1028, "queue in"=w1029) -> ("error out"=w1026:errorcluster, "queue out"=w1027:refnum<queue>)  [unwired: 2 in]
          }
        }
      }
      frame #1 {
        n308 = Wait Until Next ms Multiple(millisecond multiple=u32 200) -> ()  [unwired: 1 out]
      }
    }
    n309 = local write "Manual States"(w859) -> ()
  }
  n310 = call "Names Data Set.vi"("Name Actions"=Name_Actions."Get Names") -> ("External Sensor Names"=w45:string[])  [unwired: 1 in, 13 out]
  n311 = while {
    shift-right: [w1054] -> _
    shift-left: w48 -> [w1057]
    shift-right: [w1053] -> _
    shift-left: w47 -> [w1056]
    tunnel: w45 -> [w1050]
    tunnel: [w1049] -> w40
    tunnel: w2 -> [w1045]
    stop <- w1049 stop-if-true
    # "Gui Continuous\nUpdates"
    n312 = local read "Channel Data Tables"() -> (w1058:T16)
    n313 = Wait on Notification(notifier=w1057, timeout in ms (-1)=200, error in (no error)=w1056) -> (notifier out=w1054:refnum<notifier>, notification=w1051:T7, timed out?=w1052:bool, error out=w1053:errorcluster)  [unwired: 1 in]
    n314 = case shown="False" w1052 {
      tunnel: w1058 -> [w1081 _]
      tunnel: w1051 -> [w1077 _]
      tunnel: w1050 -> [w1079 _]
      tunnel: w1045 -> [w1066 _]
      tunnel: "<None>" ("Current Tag") -> [w1067 _]
      frame #0 {
        n315 = local read "Cartesian Type"() -> (w1074:bool)
        n316 = Unbundle By Name(w1077) -> ("LBCB Measurements"=w1078:T11[])
        n317 = case shown="\"Actuator\"" w1081 {
          tunnel: w1079 -> [_ w1091 _]
          tunnel: w1074 -> [w1085 w1090 _]
          tunnel: w1067 -> [w1084 _ w1093]
          tunnel: w1066 -> [w1082 _ _]
          frame #0 {
            w1083 = TRUE ("Include Reading")
            n318 = call "Generate Data Tables.vi"("Combined"=w1082, "Include Reading"=w1083, "Cartesian Type"=w1085, "Force Tag"=w1084, "LBCB Number"=LBCB_Number."LBCB2") -> ("Cartesian Table"=w1087:dbl[][])  [unwired: 1 in, 1 out]
            n319 = call "Generate Data Tables.vi"("Combined"=w1082, "Include Reading"=w1083, "Cartesian Type"=w1085, "Force Tag"=w1084, "LBCB Number"=LBCB_Number."LBCB1") -> ("Cartesian Table"=w1086:dbl[][])  [unwired: 1 in, 1 out]
            n320 = local write "LBCB 2 Cartesian Space"(w1087) -> ()
            n321 = local write "LBCB 1 Cartesian Space"(w1086) -> ()
          }
          frame #1 {
            n322 = call "Generate External Sensors Table.vi"("External Sensor Names"=w1091, "WithOffset"=w1090) -> ("External Sensors"=w1092:cluster{"Name":string, "Value":dbl}[])  [unwired: 1 in, 8 out]
            n323 = local write "External Sensors"(w1092) -> ()
          }
          frame #2 {
            w1094 = TRUE ("Include Reading")
            w1099 = FALSE ("Cartesian Type")
            # "Cartesian Type ignored\nbecause we are  using \nActuator Space"
            n324 = call "Generate Data Tables.vi"("Include Reading"=w1094, "Cartesian Type"=w1099, "Force Tag"=w1093, "LBCB Number"=LBCB_Number."LBCB1") -> ("Actuator Table"=w1096:dbl[][])  [unwired: 2 in, 1 out]
            n325 = call "Generate Data Tables.vi"("Include Reading"=w1094, "Cartesian Type"=w1099, "Force Tag"=w1093, "LBCB Number"=LBCB_Number."LBCB2") -> ("Actuator Table"=w1095:dbl[][])  [unwired: 2 in, 1 out]
            n326 = local write "LBCB 1 Actuator Space"(w1096) -> ()
            n327 = local write "LBCB 2 Actuator Space"(w1095) -> ()
          }
        }
        n328 = local read "Targets"() -> (w1080:T3[])
        n329 = call "Measurements 2 Target Arrays.vi"("LBCB Command Data"=w1078, "Target  Inputs"=w1080) -> ("Target  Outputs"=w1076:T3[])  [unwired: 9 in]
        n330 = local write "Mixed Mode Status"(w1077) -> ()
        n331 = call "App Parameters DAO.vi"("Actions"=Persistant_DAO_Actions."Get") -> ("Application Timing and Logging Out"=w1071:T55)  [unwired: 8 in, 2 out]
        n332 = call "Local2Global Target Values.vi"("Tag"=w1067, "Direction"=enum16{" +", " - "}." - ", "Use Offsets"=w1074, "Combined"=w1066, "AreCommands"=TRUE, "Target  Inputs"=w1076) -> ("Target  Outputs"=w1075:T3[])  [unwired: 5 in]
        n333 = Unbundle By Name(w1071) -> ("Monitor Loop.Interval"=w1069:dbl)
        n334 = local write "Current Values"(w1075) -> ()
        n335 = Multiply(x=w1069, y=1000.0) -> (x*y=w1070:dbl)
        n336 = Wait Until Next ms Multiple(millisecond multiple=w1070) -> ()  [unwired: 1 out]
      }
      frame #1 {
      }
    }
    n337 = call "NTCP Link Status DAO.vi"("DAO Actions"=DAO_Actions."Get") -> ("NTCP Link Out"=w1043:bool)  [unwired: 9 in, 1 out]
    n338 = local write "Connected"(w1043) -> ()
    n339 = local read "Typo Problem"() -> (w1048:bool)
    n340 = call "Messages.vi"() -> ("Messages"=w1047:string)  [unwired: 1 in, 10 out]
    n341 = case shown="False" w1048 {
      tunnel: w1047 -> [w1060 w1064]
      tunnel: [w1060 w1063] -> w1046
      frame #0 {
      }
      frame #1 {
        n342 = Concatenate Strings(w1064, "\r\n", "Target Typo Detected" ("string")) -> (w1063:string)
      }
    }
    n343 = local write "Messages"(w1046) -> ()
    n344 = local read "Button States"() -> (w1059:T12)
    n345 = Unbundle By Name(w1059) -> ("Exit Requested"=w1049:bool)
  }
  n346 = while {
    shift-right: [w1113] -> _
    shift-left: _ -> [w1116]
    shift-right: [w1114] -> _
    shift-left: _ -> [w1115]
    shift-right: [w1111] -> _
    shift-left: w3 -> [w1112]
    shift-right: [w1120] -> _
    shift-left: w12 -> [w1124]
    shift-right: [w1119] -> _
    shift-left: w6 -> [w1123]
    shift-right: [w1118] -> _
    shift-left: w31 -> [w1122]
    shift-right: [w1117] -> _
    shift-left: w27 -> [w1121]
    tunnel: w5 -> [w1109]
    shift-right: [w1108] -> _
    shift-left: NTCP_Mixed_Mode_States."Ntcp.Off" ("NTCP MM States") -> [w1126]
    tunnel: T26 {"NTCP commands"=enum."propose", "Transaction ID"="", "Control Point"="", "Accepted"=FALSE} ("NTCP Message") -> [w1107]
    tunnel: [w1106] -> w30
    shift-right: [w1101] -> _
    shift-left: FALSE -> [w1102]
    tunnel: w2 -> [w1100]
    stop <- w1106 stop-if-true
    # "NTCP States"
    n347 = local read "Mixed Mode Control Tabs"() -> (w1105:enum32{"Manual", "Input File", "NTCP"})
    n348 = local read "Button States"() -> (w1125:T12)
    n349 = Unbundle By Name(w1125) -> ("Auto-Start Enabled"=w1104:bool, "Auto-Accept Enabled"=w1103:bool, "Exit Requested"=w1106:bool)
    n350 = case shown="\"NTCP\"" w1105 {
      tunnel: w1126 -> [w1128 w1160]
      tunnel: [w1136 w1157] -> w1120
      tunnel: w1124 -> [w1136 w1158]
      tunnel: [w1135 w1153] -> w1119
      tunnel: w1123 -> [w1135 w1154]
      tunnel: [w1134 w1150] -> w1118
      tunnel: w1122 -> [w1134 w1151]
      tunnel: [w1133 w1148] -> w1117
      tunnel: w1121 -> [w1133 w1149]
      tunnel: [w1132 w1146] -> w1113
      tunnel: w1116 -> [w1132 w1147]
      tunnel: [w1131 w1144] -> w1114
      tunnel: w1115 -> [w1131 w1145]
      tunnel: [w1130 w1155] -> w1111
      tunnel: w1112 -> [w1130 w1156]
      tunnel: 200 ("timeout in ms (-1)") -> [_ w1159]
      tunnel: w1109 -> [_ w1152]
      tunnel: [w1128 w1143] -> w1108
      tunnel: w1107 -> [_ w1142]
      tunnel: w1104 -> [_ w1141]
      tunnel: w1103 -> [_ w1140]
      tunnel: w1102 -> [w1127 w1139]
      tunnel: [w1127 w1138] -> w1101
      tunnel: w1100 -> [_ w1137]
      frame #0 {
        n351 = Wait Until Next ms Multiple(millisecond multiple=u32 200) -> ()  [unwired: 1 out]
      }
      frame #1 {
        n352 = case shown="\"Ntcp.WaitForProposal\"" w1160 {
          selector: w1160 -> [w1168 _ w1321 w1362 w1404 _ _ _]
          tunnel: w1159 -> [w1182 w1255 w1313 w1377 w1393 w1460 w1487 _]
          tunnel: w1158 -> [w1181 w1256 w1331 w1376 w1413 w1469 w1497 w1515]
          tunnel: [w1180 w1249 w1329 w1368 w1411 w1466 w1494 w1515] -> w1157
          tunnel: w1156 -> [w1179 w1254 w1327 w1372 w1396 w1462 w1489 w1503]
          tunnel: [w1177 w1248 w1315 w1371 w1395 w1451 w1476 w1507] -> w1155
          tunnel: w1154 -> [w1176 w1263 w1330 w1367 w1412 w1449 w1491 w1520]
          tunnel: [w1174 w1260 w1328 w1367 w1410 w1448 w1491 w1509] -> w1153
          tunnel: w1152 -> [w1173 w1264 _ _ _ _ _ w1519]
          tunnel: [w1172 w1257 w1320 w1366 w1400 w1464 w1492 w1514] -> w1150
          tunnel: w1151 -> [w1172 w1257 w1320 w1366 w1400 w1465 w1493 w1514]
          tunnel: [w1171 w1258 w1319 w1365 w1408 w1467 w1495 w1513] -> w1148
          tunnel: w1149 -> [w1171 w1258 w1319 w1365 w1406 w1468 w1496 w1513]
          tunnel: [w1167 w1259 w1322 w1364 w1401 w1454 w1482 w1512] -> w1146
          tunnel: w1147 -> [w1164 w1259 w1324 w1364 w1403 w1455 w1481 w1512]
          tunnel: w1145 -> [w1163 w1270 w1318 w1378 w1397 w1459 w1486 w1511]
          tunnel: [w1166 w1268 w1317 w1373 w1398 w1458 w1485 w1511] -> w1144
          tunnel: [w1169 w1253 w1312 w1361 w1392 w1456 w1477 NTCP_Mixed_Mode_States."Ntcp.Off" ("NTCP MM States")] -> w1143
          tunnel: w1142 -> [w1165 _ w1326 _ w1402 _ _ _]
          tunnel: w1141 -> [_ _ _ _ w1388 _ _ _]
          tunnel: w1140 -> [_ _ w1307 _ _ _ _ _]
          tunnel: w1139 -> [w1162 w1244 w1306 w1356 w1387 w1452 w1484 w1506]
          tunnel: [w1161 w1244 w1306 w1356 w1387 w1452 w1484 w1506] -> w1138
          tunnel: w1137 -> [_ _ _ _ w1386 _ _ _]
          frame #0 {
            n353 = Wait on Notification(notifier=w1181, timeout in ms (-1)=w1182, error in (no error)=w1179) -> (notifier out=w1180:refnum<notifier>, notification=w1178:T35, timed out?=w1170:bool, error out=w1175:errorcluster)  [unwired: 1 in]
            n354 = case shown="False" w1170 {
              tunnel: w1178 -> [w1193 _]
              tunnel: [w1192 w1219] -> w1177
              tunnel: w1176 -> [w1191 w1220]
              tunnel: w1175 -> [w1189 w1215]
              tunnel: [w1190 w1220] -> w1174
              tunnel: w1173 -> [w1188 _]
              tunnel: [w1186 w1221] -> w1169
              tunnel: w1168 -> [_ w1221]
              tunnel: [w1185 w1218] -> w1167
              tunnel: [w1184 w1217] -> w1166
              tunnel: w1165 -> [_ w1216]
              tunnel: w1164 -> [w1185 w1211]
              tunnel: w1163 -> [w1184 w1212]
              tunnel: w1162 -> [w1183 w1214]
              tunnel: [w1183 w1213] -> w1161
              frame #0 {
                n355 = Unbundle By Name(w1193) -> ("MM Control Events"=w1187:T36)
                n356 = case shown="\"NCTP.ConnectToServer\"" w1187 {
                  tunnel: w1189 -> [w1196 w1198]
                  tunnel: [w1196 w1204] -> w1192
                  tunnel: w1191 -> [w1195 w1207]
                  tunnel: [w1195 w1206] -> w1190
                  tunnel: w1188 -> [_ w1205]
                  tunnel: [NTCP_Mixed_Mode_States."Ntcp.Off" ("NTCP MM States") NTCP_Mixed_Mode_States."Ntcp.WaitForProposal" ("NTCP MM States")] -> w1186
                  frame #0 {
                  }
                  frame #1 {
                    w1199 = TRUE ("State")
                    n357 = call "NTCP Server Change Message DAO.vi"("error in (no error)"=w1198, "NTCP Change In"=w1199, "DAO Actions"=DAO_Actions."Set") -> ("error out"=w1197:errorcluster)  [unwired: 6 in, 2 out]
                    n358 = Bundle By Name(cluster=w1205, "MM GUI Update Type"=Mixed_Mode_GUI_Update_Type."NTCP Server", "State"=w1199) -> (w1202:T31)
                    n359 = call "NoArgumentsLauncher.vi"("error in (no error)"=w1197, "Application"=NoPanelAppTypes."NTCP Socket", "Application Launcher Actions"=Launcher_Actions."Launch") -> ("error out"=w1203:errorcluster)  [unwired: 7 in, 1 out]
                    n360 = Enqueue Element(queue=w1207, element=w1202, error in (no error)=w1203) -> (queue out=w1206:refnum<queue>, error out=w1204:errorcluster)  [unwired: 1 in, 1 out]
                  }
                }
              }
              frame #1 {
                n361 = case shown="True" w1214 {
                  selector: w1214 -> [_ w1241]
                  tunnel: [w1229 w1238] -> w1219
                  tunnel: [w1227 w1239] -> w1218
                  tunnel: [w1226 w1240] -> w1217
                  tunnel: w1216 -> [w1223 _]
                  tunnel: w1215 -> [w1225 w1238]
                  tunnel: [TRUE w1241] -> w1213
                  tunnel: w1212 -> [_ w1240]
                  tunnel: w1211 -> [_ w1239]
                  frame #0 {
                    n362 = call "NTCP Network Parameters DAO.vi"("Persistent DAO Actions"=Persistant_DAO_Actions."Get") -> ("Network Parameters Out"=w1235:T60)  [unwired: 8 in, 2 out]
                    n363 = Unbundle By Name(w1235) -> ("Notification Name"=w1236:string)
                    n364 = Concatenate Strings("To " ("name (unnamed)"), w1236) -> (w1237:string)
                    "To Queue" <- w1237
                    n365 = Concatenate Strings("From " ("name (unnamed)"), w1236) -> (w1233:string)
                    "From Queue" <- w1233
                    n366 = Obtain Queue(name (unnamed)=w1237, element data type=w1223, error in (no error)=w1225) -> (queue out=w1227:refnum<queue>, error out=w1228:errorcluster)  [unwired: 2 in, 1 out]
                    n367 = Obtain Queue(name (unnamed)=w1233, element data type=T1 {"NTCP commands"=enum."propose", "Transaction ID"="", "Control Point"="", "Targets"=[]} ("NTCP Message"), error in (no error)=w1225) -> (queue out=w1226:refnum<queue>, error out=w1230:errorcluster)  [unwired: 2 in, 1 out]
                    n368 = call <vilib>:"Merge Errors.vi"("error in 3 (no error)"=w1230, "error in 2 (no error)"=w1228) -> ("error out"=w1229:errorcluster)  [unwired: 5 in]
                  }
                  frame #1 {
                  }
                }
              }
            }
          }
          frame #1 {
            n369 = Dequeue Element(queue=w1270, timeout in ms (-1)=w1255, error in (no error)=w1254) -> (queue out=w1268:refnum<queue>, element=w1269:T1, timed out?=w1245:bool, error out=w1262:errorcluster)
            "NTCP" <- w1269
            n370 = call "Monitor for NTCP Close.vi"("Skip"=Skip_NTCP_Close_Monitor."Skip NTCP", "timeout"=w1255, "error in (no error)"=w1254, "MM Button Events In"=w1256) -> ("error out"=w1247:errorcluster, "Close Received"=w1251:bool, "Button Events Out"=w1249:refnum<notifier>)  [unwired: 4 in, 1 out]
            n371 = Unbundle By Name(w1269) -> ("NTCP commands"=w1267:T2, "Transaction ID"=w1265:string, "Targets"=w1266:T3[])
            n372 = case shown="False" w1245 {
              tunnel: w1267 -> [w1279 _]
              tunnel: w1266 -> [w1278 _]
              tunnel: w1265 -> [w1277 _]
              tunnel: w1264 -> [w1276 _]
              tunnel: w1263 -> [w1275 w1304]
              tunnel: w1262 -> [w1274 w1303]
              tunnel: [w1273 w1303] -> w1261
              tunnel: [w1272 w1304] -> w1260
              tunnel: [w1271 NTCP_Mixed_Mode_States."Ntcp.WaitForProposal" ("NTCP MM States")] -> w1252
              frame #0 {
                n373 = case shown="\"propose\"" w1279 {
                  tunnel: w1278 -> [w1282 _ _]
                  tunnel: w1277 -> [w1286 _ _]
                  tunnel: w1276 -> [w1294 _ _]
                  tunnel: w1275 -> [w1296 w1299 w1301]
                  tunnel: w1274 -> [w1295 w1298 w1300]
                  tunnel: [w1289 w1298 w1300] -> w1273
                  tunnel: [w1288 w1299 w1301] -> w1272
                  tunnel: [NTCP_Mixed_Mode_States."Ntcp.WaitForAccept" ("NTCP MM States") NTCP_Mixed_Mode_States."Ntcp.WaitForProposal" ("NTCP MM States") NTCP_Mixed_Mode_States."Ntcp.Shutdown" ("NTCP MM States")] -> w1271
                  frame #0 {
                    n374 = local read "Cartesian Type"() -> (w1280:bool)
                    n375 = Bundle By Name(cluster=w1294, "MM GUI Update Type"=Mixed_Mode_GUI_Update_Type."Targets", "Targets"=w1282, "State"=w1280) -> (w1283:T31)
                    n376 = call "Extract Step Number from TransID.vi"("TransID"=w1286) -> ("Step"=w1284:string)  [unwired: 10 in]
                    n377 = Enqueue Element(queue=w1296, element=w1283, error in (no error)=w1295) -> (queue out=w1292:refnum<queue>, error out=w1290:errorcluster)  [unwired: 1 in, 1 out]
                    n378 = Bundle By Name(cluster=w1294, "MM GUI Update Type"=Mixed_Mode_GUI_Update_Type."TestStats", "Step"=w1284) -> (w1291:T31)
                    n379 = Enqueue Element(queue=w1292, element=w1291, error in (no error)=w1290) -> (queue out=w1288:refnum<queue>, error out=w1289:errorcluster)  [unwired: 1 in, 1 out]
                    n380 = call "Steps DAO.vi"("Step String In"=w1284, "Steps Actions"=T38."Set Step String") -> ()  [unwired: 7 in, 3 out]
                  }
                  frame #1 {
                  }
                  frame #2 {
                  }
                }
              }
              frame #1 {
              }
            }
            n381 = call "Can Switch Control Types.vi"("Can Switch In"=TRUE, "DAO Actions"=DAO_Actions."Set") -> ()  [unwired: 9 in, 1 out]
            n382 = call <vilib>:"Merge Errors.vi"("error in 3 (no error)"=w1261, "error in 1 (no error)"=w1247) -> ("error out"=w1248:errorcluster)  [unwired: 5 in]
            n383 = Select(t=NTCP_Mixed_Mode_States."Ntcp.Shutdown", s=w1251, f=w1252) -> (s? t:f=w1253:T21)
          }
          frame #2 {
            n384 = call "Accept Or Decline.vi"("timeout"=w1313, "error in (no error)"=w1327, "AutoAccept"=w1307, "MM Gui Updates In"=w1330, "MM Button Events In"=w1331) -> ("error out"=w1316:errorcluster, "Accepted or Declined"=w1325:T51, "MM Gui Updates Out"=w1328:refnum<queue>, "Button Events Out"=w1329:refnum<notifier>)  [unwired: 3 in]
            n385 = call "Monitor for NTCP Close.vi"("Skip"=Skip_NTCP_Close_Monitor."Skip Button Event", "timeout"=w1313, "error in (no error)"=w1316, "From NTCP In"=w1318) -> ("error out"=w1314:errorcluster, "From NTCP Out"=w1317:refnum<queue>, "Close Received"=w1310:bool)  [unwired: 4 in, 1 out]
            n386 = case shown="\"Accepted\"" w1325 {
              tunnel: w1326 -> [_ _ w1346 w1355]
              tunnel: w1324 -> [w1333 w1336 w1343 w1352]
              tunnel: w1316 -> [w1332 w1335 w1341 w1350]
              tunnel: [w1332 w1335 w1340 w1349] -> w1323
              tunnel: [w1333 w1336 w1339 w1348] -> w1322
              tunnel: [w1334 NTCP_Mixed_Mode_States."Ntcp.Shutdown" ("NTCP MM States") NTCP_Mixed_Mode_States."Ntcp.WaitForExecute" ("NTCP MM States") NTCP_Mixed_Mode_States."Ntcp.WaitForProposal" ("NTCP MM States")] -> w1311
              tunnel: w1321 -> [w1334 _ _ _]
              frame #0 {
              }
              frame #1 {
              }
              frame #2 {
                n387 = Bundle By Name(cluster=w1346, "NTCP commands"=NTCP_Commands."propose", "Accepted"=T27 TRUE) -> (w1342:T26)
                n388 = Enqueue Element(queue=w1343, element=w1342, error in (no error)=w1341) -> (queue out=w1339:refnum<queue>, error out=w1340:errorcluster)  [unwired: 1 in, 1 out]
              }
              frame #3 {
                n389 = Bundle By Name(cluster=w1355, "NTCP commands"=NTCP_Commands."propose", "Accepted"=T27 FALSE) -> (w1351:T26)
                n390 = Enqueue Element(queue=w1352, element=w1351, error in (no error)=w1350) -> (queue out=w1348:refnum<queue>, error out=w1349:errorcluster)  [unwired: 1 in, 1 out]
              }
            }
            n391 = Select(t=NTCP_Mixed_Mode_States."Ntcp.Shutdown", s=w1310, f=w1311) -> (s? t:f=w1312:T21)
            n392 = call <vilib>:"Merge Errors.vi"("error in 3 (no error)"=w1314, "error in 2 (no error)"=w1323) -> ("error out"=w1315:errorcluster)  [unwired: 5 in]
          }
          frame #3 {
            n393 = Dequeue Element(queue=w1378, timeout in ms (-1)=w1377, error in (no error)=w1372) -> (queue out=w1373:refnum<queue>, element=w1357:T1, timed out?=w1358:bool, error out=w1369:errorcluster)
            n394 = call "Monitor for NTCP Close.vi"("Skip"=Skip_NTCP_Close_Monitor."Skip NTCP", "timeout"=w1377, "error in (no error)"=w1372, "MM Button Events In"=w1376) -> ("error out"=w1370:errorcluster, "Close Received"=w1360:bool, "Button Events Out"=w1368:refnum<notifier>)  [unwired: 4 in, 1 out]
            n395 = Unbundle By Name(w1357) -> ("NTCP commands"=w1374:T2)
            n396 = local write "NTCP"(w1357) -> ()
            n397 = case shown="False" w1358 {
              tunnel: w1374 -> [w1381 _]
              tunnel: [w1380 w1385] -> w1363
              tunnel: w1362 -> [w1379 w1385]
              frame #0 {
                n398 = case shown="\"execute\"" w1381 {
                  tunnel: [w1382 NTCP_Mixed_Mode_States."Ntcp.WaitForStart" ("NTCP MM States") NTCP_Mixed_Mode_States."Ntcp.Shutdown" ("NTCP MM States")] -> w1380
                  tunnel: w1379 -> [w1382 _ _]
                  frame #0 {
                  }
                  frame #1 {
                  }
                  frame #2 {
                  }
                }
              }
              frame #1 {
              }
            }
            n399 = Select(t=NTCP_Mixed_Mode_States."Ntcp.Shutdown", s=w1360, f=w1363) -> (s? t:f=w1361:T21)
            n400 = call <vilib>:"Merge Errors.vi"("error in 2 (no error)"=w1369, "error in 1 (no error)"=w1370) -> ("error out"=w1371:errorcluster)  [unwired: 5 in]
          }
          frame #4 {
            n401 = call "Start Or Stop.vi"("timeout"=w1393, "error in (no error)"=w1396, "AutoStart"=w1388, "MM Gui Updates In"=w1412, "MM Button Events In"=w1413) -> ("error out"=w1407:errorcluster, "Start or Stop"=w1409:T51, "MM Gui Updates Out"=w1410:refnum<queue>, "Button Events Out"=w1411:refnum<notifier>)  [unwired: 3 in]
            n402 = call "Monitor for NTCP Close.vi"("Skip"=Skip_NTCP_Close_Monitor."Skip Button Event", "timeout"=w1393, "error in (no error)"=w1396, "From NTCP In"=w1397) -> ("error out"=w1394:errorcluster, "From NTCP Out"=w1398:refnum<queue>, "Close Received"=w1390:bool)  [unwired: 4 in, 1 out]
            n403 = case shown="\"No Decision Yet\"" w1409 {
              tunnel: [w1417 w1426 w1436 w1447] -> w1408
              tunnel: w1407 -> [w1416 w1422 w1432 w1446]
              tunnel: w1406 -> [w1417 w1426 w1436 w1445]
              tunnel: [w1416 w1419 w1429 w1444] -> w1405
              tunnel: [w1415 NTCP_Mixed_Mode_States."Ntcp.WaitForProposal" ("NTCP MM States") NTCP_Mixed_Mode_States."Ntcp.Shutdown" ("NTCP MM States") NTCP_Mixed_Mode_States."Ntcp.WaitForMclRamp" ("NTCP MM States")] -> w1391
              tunnel: w1404 -> [w1415 _ _ _]
              tunnel: w1403 -> [w1414 w1425 w1435 w1441]
              tunnel: w1402 -> [_ w1424 w1434 _]
              tunnel: [w1414 w1418 w1428 w1441] -> w1401
              tunnel: w1386 -> [_ _ _ w1438]
              frame #0 {
              }
              frame #1 {
                n404 = Bundle By Name(cluster=w1424, "NTCP commands"=NTCP_Commands."execute", "Accepted"=T27 FALSE) -> (w1423:T26)
                n405 = Enqueue Element(queue=w1425, element=w1423, error in (no error)=w1422) -> (queue out=w1418:refnum<queue>, error out=w1419:errorcluster)  [unwired: 1 in, 1 out]
              }
              frame #2 {
                n406 = Bundle By Name(cluster=w1434, "NTCP commands"=NTCP_Commands."execute", "Accepted"=T27 FALSE) -> (w1433:T26)
                n407 = Enqueue Element(queue=w1435, element=w1433, error in (no error)=w1432) -> (queue out=w1428:refnum<queue>, error out=w1429:errorcluster)  [unwired: 1 in, 1 out]
              }
              frame #3 {
                n408 = local read "Ramp Times"() -> (w1443:cluster{"Displacement":T15, "Force":T15})
                n409 = call "Can Switch Control Types.vi"("Can Switch In"=FALSE, "DAO Actions"=DAO_Actions."Set") -> ()  [unwired: 9 in, 1 out]
                n410 = call "Send Mixed Mode Command.vi"("MCL Command In"=w1445, "Ramp Times"=w1443, "error in"=w1446, "Combined"=w1438) -> ("MCL Command Out"=w1447:refnum<queue>, "error out"=w1444:errorcluster)  [unwired: 1 in]
              }
            }
            n411 = call <vilib>:"Merge Errors.vi"("error in 3 (no error)"=w1405, "error in 2 (no error)"=w1394) -> ("error out"=w1395:errorcluster)  [unwired: 5 in]
            n412 = Select(t=NTCP_Mixed_Mode_States."Ntcp.Shutdown", s=w1390, f=w1391) -> (s? t:f=w1392:T21)
          }
          frame #5 {
            # "Note that the ramp does not stop\nif the connection is closed"
            n413 = call "Monitor for Stop.vi"("timeout"=w1460, "error in (no error)"=w1462, "Mixed Mode Commands In"=w1468, "MM Button Events In"=w1469) -> ("error out"=w1471:errorcluster, "Mixed Mode Commands Out"=w1467:refnum<queue>, "Stop Requests"=w1470:T53, "Button Events Out"=w1466:refnum<notifier>)  [unwired: 4 in]
            n414 = call "Monitor for NTCP Close.vi"("Skip"=Skip_NTCP_Close_Monitor."Skip Button Event", "timeout"=w1460, "error in (no error)"=w1462, "From NTCP In"=w1459) -> ("error out"=w1461:errorcluster, "From NTCP Out"=w1458:refnum<queue>, "Close Received"=w1457:bool)  [unwired: 4 in, 1 out]
            n415 = call "Done Or Abort.vi"("error in (no error)"=w1462, "timeout"=w1460, "MCL State In"=w1465) -> ("error out"=w1472:errorcluster, "MCL State"=w1450:T52, "MCL State Out"=w1464:refnum<queue>)  [unwired: 1 in]
            n416 = call <vilib>:"Merge Errors.vi"("error in 3 (no error)"=w1472, "error in 2 (no error)"=w1461, "error in 1 (no error)"=w1471) -> ("error out"=w1453:errorcluster)  [unwired: 4 in]
            n417 = call "Nctp Ramp Done.vi"("Close Received"=w1457, "MCL State In"=w1450, "error in"=w1453, "Stop Requests"=w1470, "MCL Cmd In"=w1455) -> ("error out"=w1451:errorcluster, "NTCP MM Finish State"=w1456:T21, "MCL Cmd Out"=w1454:refnum<queue>)  [unwired: 2 in]
            n418 = case shown="\"Abort\"" w1450 {
              tunnel: w1449 -> [w1473 w1475]
              tunnel: [w1473 w1474] -> w1448
              frame #0 {
              }
              frame #1 {
                n419 = call "Autos Off.vi"("queue in"=w1475) -> ("queue out"=w1474:refnum<queue>)  [unwired: 3 in, 1 out]
              }
            }
          }
          frame #6 {
            n420 = call "Monitor for Stop.vi"("timeout"=w1487, "error in (no error)"=w1489, "Mixed Mode Commands In"=w1496, "MM Button Events In"=w1497) -> ("error out"=w1498:errorcluster, "Mixed Mode Commands Out"=w1495:refnum<queue>, "Stop Requests"=w1480:T53, "Button Events Out"=w1494:refnum<notifier>)  [unwired: 4 in]
            n421 = call "Monitor for NTCP Close.vi"("Skip"=Skip_NTCP_Close_Monitor."Skip Button Event", "timeout"=w1487, "error in (no error)"=w1489, "From NTCP In"=w1486) -> ("error out"=w1488:errorcluster, "From NTCP Out"=w1485:refnum<queue>, "Close Received"=w1478:bool)  [unwired: 4 in, 1 out]
            n422 = call "MCL Ramping.vi"("error in (no error)"=w1489, "timeout"=w1487, "MCL State In"=w1493) -> ("error out"=w1499:errorcluster, "Is Ramping?"=w1479:bool, "MCL State Out"=w1492:refnum<queue>)  [unwired: 1 in]
            n423 = call <vilib>:"Merge Errors.vi"("error in 3 (no error)"=w1499, "error in 2 (no error)"=w1488, "error in 1 (no error)"=w1498) -> ("error out"=w1483:errorcluster)  [unwired: 4 in]
            n424 = call "Nctp Ramp Running.vi"("Close Received"=w1478, "MCL Ramp Running?"=w1479, "error in"=w1483, "Stop Requests"=w1480, "MCL Cmd In"=w1481) -> ("error out"=w1476:errorcluster, "NTCP MM Finish State"=w1477:T21, "MCL Cmd Out"=w1482:refnum<queue>)  [unwired: 2 in]
          }
          frame #7 {
            w1501 = FALSE ("State")
            # "Need to send an app event"
            n425 = Bundle By Name(cluster=w1519, "MM GUI Update Type"=Mixed_Mode_GUI_Update_Type."NTCP Server", "State"=w1501) -> (w1517:T31)
            n426 = call "NTCP Server Change Message DAO.vi"("error in (no error)"=w1503, "NTCP Change In"=w1501, "DAO Actions"=DAO_Actions."Set") -> ("error out"=w1500:errorcluster)  [unwired: 6 in, 2 out]
            n427 = call "Can Switch Control Types.vi"("Can Switch In"=TRUE, "DAO Actions"=DAO_Actions."Set") -> ()  [unwired: 9 in, 1 out]
            n428 = Enqueue Element(queue=w1520, element=w1517, error in (no error)=w1500) -> (queue out=w1510:refnum<queue>, error out=w1508:errorcluster)  [unwired: 1 in, 1 out]
            n429 = call "Autos Off.vi"("error in"=w1508, "queue in"=w1510) -> ("error out"=w1507:errorcluster, "queue out"=w1509:refnum<queue>)  [unwired: 2 in]
          }
        }
      }
    }
    "NTCP MM States" <- w1108
  }
  n430 = while {
    shift-right: [w1532] -> _
    shift-left: w19 -> [w1540]
    shift-right: [w1536] -> _
    shift-left: w44 -> [w1541]
    shift-right: [w1533] -> _
    shift-left: w31 -> [w1535]
    shift-right: [w1531] -> _
    shift-left: _ -> [w1530]
    tunnel: [w1528] -> w39
    shift-right: [w1523] -> _
    shift-left: w18 -> [w1524]
    tunnel: w17 -> [w1521]
    stop <- w1528 stop-if-true
    # "Master Control Loop\nState Monitor"
    n431 = Dequeue Element(queue=w1541, timeout in ms (-1)=200, error in (no error)=w1540) -> (queue out=w1536:refnum<queue>, element=w1537:T9, timed out?=w1538:bool, error out=w1534:errorcluster)
    n432 = call "Fault List 2 Indicators.vi"("Use LBCB Selector"=FALSE) -> ("Forces"=w1525:bool, "Displacement"=w1526:bool, "Increments"=w1522:bool)  [unwired: 7 in, 1 out]
    n433 = case shown="False" w1538 {
      tunnel: w1537 -> [w1542 _]
      tunnel: w1535 -> [w1557 w1592]
      tunnel: w1534 -> [w1548 w1591]
      tunnel: [w1556 w1592] -> w1533
      tunnel: [w1555 w1591] -> w1532
      tunnel: [w1551 w1593] -> w1531
      tunnel: w1530 -> [w1552 w1593]
      tunnel: w1524 -> [w1550 w1590]
      tunnel: [w1549 w1590] -> w1523
      tunnel: w1521 -> [w1546 _]
      frame #0 {
        n434 = local read "Test Statistics"() -> (w1544:cluster{"Steps":string, "Elapsed \nTime":dbl})
        n435 = call "States 2 Leds.vi"("MixedModeStates"=w1542) -> ("Mixed Mode State Display"=w1554:T23)  [unwired: 10 in]
        n436 = Unbundle By Name(w1544) -> ("Steps"=w1543:string)
        n437 = case shown="\"Start Initial Ramp\"" w1542 {
          tunnel: [MCL_States."MCL Idle" ("notification") MCL_States."MCL Idle" ("notification") MCL_States."MCL Idle" ("notification") MCL_States."MCL Idle" ("notification") MCL_States."MCL Idle" ("notification") MCL_States."MCL Ramping" ("notification") MCL_States."MCL Ramping" ("notification") MCL_States."MCL Ramping" ("notification") MCL_States."MCL Ramping" ("notification") MCL_States."MCL Ramping" ("notification") MCL_States."MCL Ramping" ("notification") MCL_States."MCL Ramping" ("notification") MCL_States."MCL Ramping" ("notification") MCL_States."MCL Ramping" ("notification") MCL_States."MCL Ramping" ("notification") MCL_States."MCL Ramping" ("notification") MCL_States."MCL Ramping" ("notification") MCL_States."MCL Holding" ("notification") MCL_States."MCL Holding" ("notification") MCL_States."MCL Holding" ("notification") MCL_States."MCL Holding" ("notification") MCL_States."MCL Done" ("notification") MCL_States."MCL Aborting" ("notification") MCL_States."MCL Done" ("notification") MCL_States."MCL Idle" ("notification")] -> w1551
          frame #0 {
          }
          frame #1 {
          }
          frame #2 {
          }
          frame #3 {
          }
          frame #4 {
          }
          frame #5 {
          }
          frame #6 {
          }
          frame #7 {
          }
          frame #8 {
          }
          frame #9 {
          }
          frame #10 {
          }
          frame #11 {
          }
          frame #12 {
          }
          frame #13 {
          }
          frame #14 {
          }
          frame #15 {
          }
          frame #16 {
          }
          frame #17 {
          }
          frame #18 {
          }
          frame #19 {
          }
          frame #20 {
          }
          frame #21 {
          }
          frame #22 {
          }
          frame #23 {
          }
          frame #24 {
          }
        }
        n438 = Bundle By Name(cluster=w1546, "Step"=w1543, "MixedModeStates"=w1542) -> (w1545:T25)
        n439 = local write "Mixed Mode State Display"(w1554) -> ()
        n440 = Enqueue Element(queue=w1550, element=w1545, error in (no error)=w1548) -> (queue out=w1549:refnum<queue>, error out=w1547:errorcluster)  [unwired: 1 in, 1 out]
        n441 = Not Equal?(x=w1551, y=w1552) -> (x != y?=w1553:bool)
        n442 = case shown="False" w1553 {
          tunnel: w1557 -> [w1559 w1564]
          tunnel: w1547 -> [w1558 w1563]
          tunnel: [w1559 w1562] -> w1556
          tunnel: [w1558 w1561] -> w1555
          tunnel: w1551 -> [_ w1560]
          frame #0 {
          }
          frame #1 {
            n443 = Enqueue Element(queue=w1564, element=w1560, error in (no error)=w1563) -> (queue out=w1562:refnum<queue>, error out=w1561:errorcluster)  [unwired: 1 in, 1 out]
          }
        }
        n444 = local write "MCL States"(w1551) -> ()
      }
      frame #1 {
      }
    }
    n445 = local write "Displacement Limit"(w1526) -> ()
    n446 = local write "Force Limit"(w1525) -> ()
    n447 = local write "Increment Limit"(w1522) -> ()
    n448 = local read "Button States"() -> (w1529:T12)
    n449 = Unbundle By Name(w1529) -> ("Exit Requested"=w1528:bool)
  }
  n450 = Compound Arithmetic op=AND(w56, w55, w52, w40, w36, w39, w35, w30) -> (w62:bool)
  n451 = Not(x=w62) -> (.not. x?=w61:bool)
  n452 = flat-sequence {
    tunnel: w61 -> [w1596]
    tunnel: [w1596] -> w60
    frame #0 {
      n453 = control-ref of="This VI"() -> (w1595:refnum<vi>)
      n454 = property class="VI"(reference=w1595, "Front Panel.Open"=FALSE ("Front Panel Window:Open")) -> ()  [unwired: 1 in, 2 out]
    }
  }
  n455 = local write "App Stop"(w60) -> ()
